vi "DblMonoPMDCurrentScanSM correction.vi"() -> ()   [LabVIEW 2009]
uses:
  <vilib>/DAQmx/create/channels.llb/DAQmx Create Channel (AI-Voltage-Basic).vi
  <vilib>/DAQmx/create/channels.llb/DAQmx Create Channel (AO-Voltage-Basic).vi
  <vilib>/DAQmx/write.llb/DAQmx Write (Analog DBL 1Chan 1Samp).vi
  <vilib>/DAQmx/read.llb/DAQmx Read (Analog 1D DBL 1Chan NSamp).vi
  <vilib>/DAQmx/configure/timing.llb/DAQmx Timing (Sample Clock).vi
  <vilib>/DAQmx/read.llb/DAQmx Read (Analog 1D DBL NChan 1Samp).vi
  <vilib>/DAQmx/write.llb/DAQmx Write (Analog 2D DBL NChan NSamp).vi
  <vilib>/Utility/file.llb/Write To Spreadsheet File (DBL).vi
  <vilib>/Analysis/NI_AALBase.lvlib
panel:
  in  "Volts/pixel":dbl
  out "Xin":dbl
  out "Yin":dbl
  in  "Correction":dbl[][](array[numeric])
  in  "Scan mirrors out":tag
  in  "Scan Mirrors in":tag
  in  "Voltage B":dbl min=-10.0 max=10.0 step=0.1 format="%0.2f"
  in  "Voltage A":dbl min=-10.0 max=10.0 step=0.1 format="%0.2f"
  in  "Output B":tag="Dev1/ao3"
  in  "Output A":tag="Dev1/ao2"
  in  "Input Channel":tag="Dev1/ai6"
  in  "Current":bool
  in  "Power":bool=TRUE
  out "ScanGraph":cluster{dbl[], dbl[]}(graph)
  in  "Sensitivity":dbl=1e-09 caption="(A/V)" format="%#_6p"
  out "Readout":dbl=-2.45576047e-07 format="%^#_9e"
  in  "Scan Save Path":path
  in  "On":bool=TRUE
  out "Waveform Chart":dbl(graph)=-2.45576047e-07
  in  "Save":bool=TRUE
  in  "Exit":bool
  in  "STOP":bool
  in  "Step Time (sec)":dbl=1.0 min=0.001 max=300.0 step=0.001 format="%.3f"
  in  "Step Size (nm)":dbl=1.0 min=0.1 max=100.0 step=0.1 format="%.1f"
  in  "End":dbl=800.0 min=0.0 max=2000.0 step=0.1 format="%.1f"
  in  "Start":dbl=400.0 min=0.0 max=2000.0 step=0.1 format="%.1f"
  in  "Scan":bool
  in  "Up":bool=TRUE caption="Down"
  in  "Increment (nm)":dbl=10.0 min=0.1 max=2000.0 step=0.1 format="%.1f"
  in  "PMD Settings":T1={"Beam Diameter (mm)"=4.0, "BWIn"=0, "Averaging Rate"=300, "Auto Range"=TRUE} {"Averaging Rate" min=33 max=5000 step=1; "BWIn" items=["HIGH", "LOW"]; "Beam Diameter (mm)" min=1.0 max=9.0 step=0.5}
  in  "Step":bool
  out "Busy":bool=TRUE
  in  "Send Command":bool
  in  "Command":u16(ring)=1 items=["nm", "goto", "nm/min", "VIS grating", "IR grating"]
  in  "Wavelength (nm)":dbl=500.0 min=0.0 max=2000.0 step=0.1 format="%.1f"
  in  "Scan Speed (nm/min)":dbl=100.0 min=1.0 max=500.0 step=0.1 format="%.1f"
  out "Done?":string="   ..."
  in  "Send Question":bool
  in  "Ask?":u16(ring) items=["?nm", "?nm/min", "?grating", "?turret", "?gratings"]
  in  "Zero?":bool
  out "PM Error log":string="-222,\"Data out of range\"\n-222,\"Data out of range\"\n-222,\"Data out of range\"\n-222,\"Data out of range\"\n-222,\"Data out of range\"\n-222,\"Data out of range\"\n-222,\"Data out of range\"\n-222,\"Data out of range\"\n-222,\"Data out of range\"\n-222,\"Data out of range\"\n-222,\"Data out of range\"\n-222,\"Data out of range\"\n-222,\"Data out of range\"\n-222,\"Data out of range\"\n-222,\"Data out of range\"\n-222,\"Data out of range\"\n-222,\"Data out of range\"\n-222,\"Data out of range\"\n-222,\"Data out of range\"\n-222,\"Data out of range\"\n-222,\"Data out of range\"\n-222,\"Data out of range\"\n-222,\"Data out of range\"\n-222,\"Data out of range\"\n-222,\"Data out of range\"\n-222,\"Data out of range\"\n-222,\"Data out of range\"\n-222,\"Data out of range\"\n-222,\"Data out of range\"\n-222,\"Data out of range\"\n-222,\"Data out of range\"\n-222,\"Data out of range\"\n-222,\"Data out of range\"\n-222,\"Data out of range\"\n-222,\"Data out of range\"\n-222,\"Data out of range\"\n-222,\"Data out of range\"\n-222,\"Data out of range\"\n-222,\"Data out of range\"\n-222,\"Data out of range\"\n-222,\"Data out of range\"\n-222,\"Data out of range\"\n-222,\"Data out of range\"\n-222,\"Data out of range\"\n-222,\"Data out of range\"\n-222,\"Data out of range\"\n-222,\"Data out of range\"\n-222,\"Data out of range\"\n-222,\"Data out of range\"\n-222,\"Data out of range\"\n-222,\"Data out of range\"\n-222,\"Data out of range\"\n-222,\"Data out of range\"\n-222,\"Data out of range\"\n-222,\"Data out of range\"\n-222,\"Data out of range\"\n-222,\"Data out of range\"\n-222,\"Data out of range\"\n-222,\"Data out of range\"\n-222,\"Data out of range\"\n-222,\"Data out of range\"\n-222,\"Data out of range\"\n-222,\"Data out of range\"\n-222,\"Data out of range\"\n-222,\"Data out of range\"\n-222,\"Data out of range\"\n-222,\"Data out of range\"\n-222,\"Data out of range\"\n-222,\"Data out of range\"\n-222,\"Data out of range\"\n-222,\"Data out of range\"\n-222,\"Data out of range\"\n-222,\"Data out of range\"\n-222,\"Data out of range\"\n-222,\"Data out of range\"\n-222,\"Data out of range\"\n-222,\"Data out of range\"\n-222,\"Data out of range\"\n-222,\"Data out of range\"\n-222,\"Data out of range\"\n-222,\"Data out of range\"\n-222,\"Data out of range\"\n-222,\"Data out of range\"\n-222,\"Data out of range\"\n-222,\"Data out of range\"\n-222,\"Data out of range\"\n-222,\"Data out of range\"\n-222,\"Data out of range\"\n-222,\"Data out of range\"\n-222,\"Data out of range\"\n-222,\"Data out of range\"\n-222,\"Data out of range\"\n-222,\"Data out of range\"\n-222,\"Data out of range\"\n-222,\"Data out of range\"\n-222,\"Data out of range\"\n-222,\"Data out of range\"\n-222,\"Data out of range\"\n-222,\"Data out of range\"\n-222,\"Data out of range\"\n-222,\"Data out of range\"\n-222,\"Data out of range\"\n-222,\"Data out of range\"\n-222,\"Data out of range\"\n-222,\"Data out of range\"\n-222,\"Data out of range\"\n-222,\"Data out of range\"\n-222,\"Data out of range\"\n-222,\"Data out of range\"\n-222,\"Data out of range\"\n-222,\"Data out of range\"\n-222,\"Data out of range\"\n-222,\"Data out of range\"\n-222,\"Data out of range\"\n-222,\"Data out of range\"\n-222,\"Data out of range\"\n-222,\"Data out of range\"\n-222,\"Data out of range\"\n-222,\"Data out of range\"\n-222,\"Data out of range\"\n-222,\"Data out of range\"\n-222,\"Data out of range\"\n-222,\"Data out of range\"\n-222,\"Data out of range\"\n-222,\"Data out of range\"\n-222,\"Data out of range\"\n-222,\"Data out of range\"\n-222,\"Data out of range\"\n-222,\"Data out of range\"\n-222,\"Data out of range\"\n-222,\"Data out of range\"\n-222,\"Data out of range\"\n-222,\"Data out of range\"\n-222,\"Data out of range\"\n-222,\"Data out of range\"\n-222,\"Data out of range\"\n-222,\"Data out of range\"\n-222,\"Data out of range\"\n-222,\"Data out of range\"\n-222,\"Data out of range\"\n-222,\"Data out of range\"\n-222,\"Data out of range\"\n-222,\"Data out of range\"\n-222,\"Data out of range\"\n-222,\"Data out of range\"\n-222,\"Data out of range\"\n-222,\"Data out of range\"\n-222,\"Data out of range\"\n-222,\"Data out of range\"\n-222,\"Data out of range\"\n-222,\"Data out of range\"\n-222,\"Data out of range\"\n-222,\"Data out of range\"\n-222,\"Data out of range\"\n-222,\"Data out of range\"\n-222,\"Data out of range\"\n-222,\"Data out of range\"\n-222,\"Data out of range\"\n-222,\"Data out of range\"\n-222,\"Data out of range\"\n-222,\"Data out of range\"\n-222,\"Data out of range\"\n-222,\"Data out of range\"\n-222,\"Data out of range\"\n-222,\"Data out of range\"\n-222,\"Data out of range\"\n-222,\"Data out of range\"\n-222,\"Data out of range\"\n-222,\"Data out of range\"\n-222,\"Data out of range\"\n-222,\"Data out of range\"\n-222,\"Data out of range\"\n-222,\"Data out of range\"\n-222,\"Data out of range\"\n-222,\"Data out of range\"\n-222,\"Data out of range\"\n-222,\"Data out of range\"\n-222,\"Data out of range\"\n-222,\"Data out of range\"\n-222,\"Data out of range\"\n-222,\"Data out of range\"\n-222,\"Data out of range\"\n-222,\"Data out of range\"\n-222,\"Data out of range\"\n-222,\"Data out of range\"\n-222,\"Data out of range\"\n-222,\"Data out of range\"\n-222,\"Data out of range\"\n-222,\"Data out of range\"\n-222,\"Data out of range\"\n-222,\"Data out of range\"\n-222,\"Data out of range\"\n-222,\"Data out of range\"\n-222,\"Data out of range\"\n-222,\"Data out of range\"\n-222,\"Data out of range\"\n-222,\"Data out of range\"\n-222,\"Data out of range\"\n-222,\"Data out of range\"\n-222,\"Data out of range\"\n-222,\"Data out of range\"\n-222,\"Data out of range\"\n-222,\"Data out of range\"\n-222,\"Data out of range\"\n-222,\"Data out of range\"\n-222,\"Data out of range\"\n-222,\"Data out of range\"\n-222,\"Data out of range\"\n-222,\"Data out of range\"\n-222,\"Data out of range\"\n-222,\"Data out of range\"\n-222,\"Data out of range\"\n-222,\"Data out of range\"\n-222,\"Data out of range\"\n-222,\"Data out of range\"\n-222,\"Data out of range\"\n-222,\"Data out of range\"\n-222,\"Data out of range\"\n-222,\"Data out of range\"\n-222,\"Data out of range\"\n-222,\"Data out of range\"\n-222,\"Data out of range\"\n-222,\"Data out of range\"\n-222,\"Data out of range\"\n-222,\"Data out of range\"\n-222,\"Data out of range\"\n-222,\"Data out of range\"\n-222,\"Data out of range\"\n-222,\"Data out of range\"\n-222,\"Data out of range\"\n-222,\"Data out of range\"\n-222,\"Data out of range\"\n-222,\"Data out of range\"\n-222,\"Data out of range\"\n-222,\"Data out of range\"\n-222,\"Data out of range\"\n-222,\"Data out of range\"\n-222,\"Data out of range\"\n-222,\"Data out of range\"\n-222,\"Data out of range\"\n-222,\"Data out of range\"\n-222,\"Data out of range\"\n-222,\"Data out of range\"\n-222,\"Data out of range\"\n-222,\"Data out of range\"\n-222,\"Data out of range\"\n-222,\"Data out of range\"\n-222,\"Data out of range\"\n-222,\"Data out of range\"\n-222,\"Data out of range\"\n-222,\"Data out of range\"\n-222,\"Data out of range\"\n-222,\"Data out of range\"\n-222,\"Data out of range\"\n-222,\"Data out of range\"\n-222,\"Data out of range\"\n-222,\"Data out of range\"\n-222,\"Data out of range\"\n-222,\"Data out of range\"\n-222,\"Data out of range\"\n-222,\"Data out of range\"\n-222,\"Data out of range\"\n-222,\"Data out of range\"\n-222,\"Data out of range\"\n-222,\"Data out of range\"\n-222,\"Data out of range\"\n-222,\"Data out of range\"\n-222,\"Data out of range\"\n-222,\"Data out of range\"\n-222,\"Data out of range\"\n-222,\"Data out of range\"\n-222,\"Data out of range\"\n-222,\"Data out of range\"\n-222,\"Data out of range\"\n-222,\"Data out of range\"\n-222,\"Data out of range\"\n-222,\"Data out of range\"\n-222,\"Data out of range\"\n-222,\"Data out of range\"\n-222,\"Data out of range\"\n-222,\"Data out of range\"\n-222,\"Data out of range\"\n-222,\"Data out of range\"\n-222,\"Data out of range\"\n-222,\"Data out of range\"\n-222,\"Data out of range\"\n-222,\"Data out of range\"\n-222,\"Data out of range\"\n-222,\"Data out of range\"\n-222,\"Data out of range\"\n-222,\"Data out of range\"\n-222,\"Data out of range\"\n-222,\"Data out of range\"\n-222,\"Data out of range\"\n-222,\"Data out of range\"\n-222,\"Data out of range\"\n-222,\"Data out of range\"\n-222,\"Data out of range\"\n-222,\"Data out of range\"\n-222,\"Data out of range\"\n-222,\"Data out of range\"\n-222,\"Data out of range\"\n-222,\"Data out of range\"\n-222,\"Data out of range\"\n-222,\"Data out of range\"\n-222,\"Data out of range\"\n-222,\"Data out of range\"\n-222,\"Data out of range\"\n-222,\"Data out of range\"\n-222,\"Data out of range\"\n-222,\"Data out of range\"\n-222,\"Data out of range\"\n-222,\"Data out of range\"\n-222,\"Data out of range\"\n-222,\"Data out of range\"\n-222,\"Data out of range\"\n-222,\"Data out of range\"\n-222,\"Data out of range\"\n-222,\"Data out of range\"\n-222,\"Data out of range\"\n-222,\"Data out of range\"\n-222,\"Data out of range\"\n-222,\"Data out of range\"\n-222,\"Data out of range\"\n-222,\"Data out of range\"\n-222,\"Data out of range\"\n-222,\"Data out of range\"\n-222,\"Data out of range\"\n-222,\"Data out of range\"\n-222,\"Data out of range\"\n-222,\"Data out of range\"\n-222,\"Data out of range\"\n-222,\"Data out of range\"\n-222,\"Data out of range\"\n-222,\"Data out of range\"\n-222,\"Data out of range\"\n-222,\"Data out of range\"\n-222,\"Data out of range\"\n-222,\"Data out of range\"\n-222,\"Data out of range\"\n-222,\"Data out of range\"\n-222,\"Data out of range\"\n-222,\"Data out of range\"\n-222,\"Data out of range\"\n-222,\"Data out of range\"\n-222,\"Data out of range\"\n-222,\"Data out of range\"\n-222,\"Data out of range\"\n-222,\"Data out of range\"\n-222,\"Data out of range\"\n-222,\"Data out of range\"\n-222,\"Data out of range\"\n-222,\"Data out of range\"\n-222,\"Data out of range\"\n-222,\"Data out of range\"\n-222,\"Data out of range\"\n-222,\"Data out of range\"\n-222,\"Data out of range\"\n-222,\"Data out of range\"\n-222,\"Data out of range\"\n-222,\"Data out of range\"\n-222,\"Data out of range\"\n-222,\"Data out of range\"\n-222,\"Data out of range\"\n-222,\"Data out of range\"\n-222,\"Data out of range\"\n-222,\"Data out of range\"\n-222,\"Data out of range\"\n-222,\"Data out of range\"\n-222,\"Data out of range\"\n-222,\"Data out of range\"\n-222,\"Data out of range\"\n-222,\"Data out of range\"\n-222,\"Data out of range\"\n-222,\"Data out of range\"\n-222,\"Data out of range\"\n-222,\"Data out of range\"\n-222,\"Data out of range\"\n-222,\"Data out of range\"\n-222,\"Data out of range\"\n-222,\"Data out of range\"\n-222,\"Data out of range\"\n-222,\"Data out of range\"\n-222,\"Data out of range\"\n-222,\"Data out of range\"\n-222,\"Data out of range\"\n-222,\"Data out of range\"\n-222,\"Data out of range\"\n-222,\"Data out of range\"\n-222,\"Data out of range\"\n-222,\"Data out of range\"\n-222,\"Data out of range\"\n-222,\"Data out of range\"\n-222,\"Data out of range\"\n-222,\"Data out of range\"\n-222,\"Data out of range\"\n-222,\"Data out of range\"\n-222,\"Data out of range\"\n-222,\"Data out of range\"\n-222,\"Data out of range\"\n-222,\"Data out of range\"\n-222,\"Data out of range\"\n-222,\"Data out of range\"\n-222,\"Data out of range\"\n-222,\"Data out of range\"\n-222,\"Data out of range\"\n-222,\"Data out of range\"\n-222,\"Data out of range\"\n-222,\"Data out of range\"\n-222,\"Data out of range\"\n-222,\"Data out of range\"\n-222,\"Data out of range\"\n-222,\"Data out of range\"\n-222,\"Data out of range\"\n-222,\"Data out of range\"\n-222,\"Data out of range\"\n-222,\"Data out of range\"\n-222,\"Data out of range\"\n-222,\"Data out of range\"\n-222,\"Data out of range\"\n-222,\"Data out of range\"\n-222,\"Data out of range\"\n-222,\"Data out of range\"\n-222,\"Data out of range\"\n-222,\"Data out of range\"\n-222,\"Data out of range\"\n-222,\"Data out of range\"\n-222,\"Data out of range\"\n-222,\"Data out of range\"\n-222,\"Data out of range\"\n-222,\"Data out of range\"\n-222,\"Data out of range\"\n-222,\"Data out of range\"\n-222,\"Data out of range\"\n-222,\"Data out of range\"\n-222,\"Data out of range\"\n-222,\"Data out of range\"\n-222,\"Data out of range\"\n-222,\"Data out of range\"\n-222,\"Data out of range\"\n-222,\"Data out of range\"\n-222,\"Data out of range\"\n-222,\"Data out of range\"\n-222,\"Data out of range\"\n-222,\"Data out of range\"\n-222,\"Data out of range\"\n-222,\"Data out of range\"\n-222,\"Data out of range\"\n-222,\"Data out of range\"\n-222,\"Data out of range\"\n-222,\"Data out of range\"\n-222,\"Data out of range\"\n-222,\"Data out of range\"\n-222,\"Data out of range\"\n-222,\"Data out of range\"\n-222,\"Data out of range\"\n-222,\"Data out of range\"\n-222,\"Data out of range\"\n-222,\"Data out of range\"\n-222,\"Data out of range\"\n-222,\"Data out of range\"\n-222,\"Data out of range\"\n-222,\"Data out of range\"\n-222,\"Data out of range\"\n-222,\"Data out of range\"\n-222,\"Data out of range\"\n-222,\"Data out of range\"\n-222,\"Data out of range\"\n-222,\"Data out of range\"\n-222,\"Data out of range\"\n-222,\"Data out of range\"\n-222,\"Data out of range\"\n-222,\"Data out of range\"\n-222,\"Data out of range\"\n-222,\"Data out of range\"\n-222,\"Data out of range\"\n-222,\"Data out of range\"\n-222,\"Data out of range\"\n-222,\"Data out of range\"\n-222,\"Data out of range\"\n-222,\"Data out of range\"\n-222,\"Data out of range\"\n-222,\"Data out of range\"\n-222,\"Data out of range\"\n-222,\"Data out of range\"\n-222,\"Data out of range\"\n-222,\"Data out of range\"\n-222,\"Data out of range\"\n-222,\"Data out of range\"\n-222,\"Data out of range\"\n-222,\"Data out of range\"\n-222,\"Data out of range\"\n-222,\"Data out of range\"\n-222,\"Data out of range\"\n-222,\"Data out of range\"\n-222,\"Data out of range\"\n-222,\"Data out of range\"\n-222,\"Data out of range\"\n-222,\"Data out of range\"\n-222,\"Data out of range\"\n-222,\"Data out of range\"\n-222,\"Data out of range\"\n-222,\"Data out of range\"\n-222,\"Data out of range\"\n-222,\"Data out of range\"\n-222,\"Data out of range\"\n-222,\"Data out of range\"\n-222,\"Data out of range\"\n-222,\"Data out of range\"\n-222,\"Data out of range\"\n-222,\"Data out of range\"\n-222,\"Data out of range\"\n-222,\"Data out of range\"\n-222,\"Data out of range\"\n-222,\"Data out of range\"\n-222,\"Data out of range\"\n-222,\"Data out of range\"\n-222,\"Data out of range\"\n-222,\"Data out of range\"\n-222,\"Data out of range\"\n-222,\"Data out of range\"\n-222,\"Data out of range\"\n-222,\"Data out of range\"\n-222,\"Data out of range\"\n-222,\"Data out of range\"\n-222,\"Data out of range\"\n-222,\"Data out of range\"\n-222,\"Data out of range\"\n-222,\"Data out of range\"\n-222,\"Data out of range\"\n-222,\"Data out of range\"\n-222,\"Data out of range\"\n-222,\"Data out of range\"\n-222,\"Data out of range\"\n-222,\"Data out of range\"\n-222,\"Data out of range\"\n-222,\"Data out of range\"\n-222,\"Data out of range\"\n-222,\"Data out of range\"\n-222,\"Data out of range\"\n-222,\"Data out of range\"\n-222,\"Data out of range\"\n-222,\"Data out of range\"\n-222,\"Data out of range\"\n-222,\"Data out of range\"\n-222,\"Data out of range\"\n-222,\"Data out of range\"\n-222,\"Data out of range\"\n-222,\"Data out of range\"\n-222,\"Data out of range\"\n-222,\"Data out of range\"\n-222,\"Data out of range\"\n-222,\"Data out of range\"\n-222,\"Data out of range\"\n-222,\"Data out of range\"\n-222,\"Data out of range\"\n-222,\"Data out of range\"\n-222,\"Data out of range\"\n-222,\"Data out of range\"\n-222,\"Data out of range\"\n-222,\"Data out of range\"\n-222,\"Data out of range\"\n-222,\"Data out of range\"\n-222,\"Data out of range\"\n-222,\"Data out of range\"\n-222,\"Data out of range\"\n-222,\"Data out of range\"\n-222,\"Data out of range\"\n-222,\"Data out of range\"\n-222,\"Data out of range\"\n-222,\"Data out of range\"\n-222,\"Data out of range\"\n-222,\"Data out of range\"\n-222,\"Data out of range\"\n-222,\"Data out of range\"\n-222,\"Data out of range\"\n-222,\"Data out of range\"\n-222,\"Data out of range\"\n-222,\"Data out of range\"\n-222,\"Data out of range\"\n-222,\"Data out of range\"\n-222,\"Data out of range\"\n-222,\"Data out of range\"\n-222,\"Data out of range\"\n-222,\"Data out of range\"\n-222,\"Data out of range\"\n-222,\"Data out of range\"\n-222,\"Data out of range\"\n-222,\"Data out of range\"\n-222,\"Data out of range\"\n-222,\"Data out of range\"\n-222,\"Data out of range\"\n-222,\"Data out of range\"\n-222,\"Data out of range\"\n-222,\"Data out of range\"\n-222,\"Data out of range\"\n-222,\"Data out of range\"\n-222,\"Data out of range\"\n-222,\"Data out of range\"\n-222,\"Data out of range\"\n-222,\"Data out of range\"\n-222,\"Data out of range\"\n-222,\"Data out of range\"\n-222,\"Data out of range\"\n-222,\"Data out of range\"\n-222,\"Data out of range\"\n-222,\"Data out of range\"\n-222,\"Data out of range\"\n-222,\"Data out of range\"\n-222,\"Data out of range\"\n-222,\"Data out of range\"\n-222,\"Data out of range\"\n-222,\"Data out of range\"\n-222,\"Data out of range\"\n-222,\"Data out of range\"\n-222,\"Data out of range\"\n-222,\"Data out of range\"\n-222,\"Data out of range\"\n-222,\"Data out of range\"\n-222,\"Data out of range\"\n-222,\"Data out of range\"\n-222,\"Data out of range\"\n-222,\"Data out of range\"\n-222,\"Data out of range\"\n-222,\"Data out of range\"\n-222,\"Data out of range\"\n-222,\"Data out of range\"\n-222,\"Data out of range\"\n-222,\"Data out of range\"\n-222,\"Data out of range\"\n-222,\"Data out of range\"\n-222,\"Data out of range\"\n-222,\"Data out of range\"\n-222,\"Data out of range\"\n-222,\"Data out of range\"\n-222,\"Data out of range\"\n-222,\"Data out of range\"\n-222,\"Data out of range\"\n-222,\"Data out of range\"\n-222,\"Data out of range\"\n-222,\"Data out of range\"\n-222,\"Data out of range\"\n-222,\"Data out of range\"\n-222,\"Data out of range\"\n-222,\"Data out of range\"\n-222,\"Data out of range\"\n-222,\"Data out of range\"\n-222,\"Data out of range\"\n-222,\"Data out of range\"\n-222,\"Data out of range\"\n-222,\"Data out of range\"\n-222,\"Data out of range\"\n-222,\"Data out of range\"\n-222,\"Data out of range\"\n-222,\"Data out of range\"\n-222,\"Data out of range\"\n-222,\"Data out of range\"\n-222,\"Data out of range\"\n-222,\"Data out of range\"\n-222,\"Data out of range\"\n-222,\"Data out of range\"\n-222,\"Data out of range\"\n-222,\"Data out of range\"\n-222,\"Data out of range\"\n-222,\"Data out of range\"\n-222,\"Data out of range\"\n-222,\"Data out of range\"\n-222,\"Data out of range\"\n-222,\"Data out of range\"\n-222,\"Data out of range\"\n-222,\"Data out of range\"\n-222,\"Data out of range\"\n-222,\"Data out of range\"\n-222,\"Data out of range\"\n-222,\"Data out of range\"\n-222,\"Data out of range\"\n-222,\"Data out of range\"\n-222,\"Data out of range\"\n-222,\"Data out of range\"\n-222,\"Data out of range\"\n-222,\"Data out of range\"\n-222,\"Data out of range\"\n-222,\"Data out of range\"\n-222,\"Data out of range\"\n-222,\"Data out of range\"\n-222,\"Data out of range\"\n-222,\"Data out of range\"\n-222,\"Data out of range\"\n-222,\"Data out of range\"\n-222,\"Data out of range\"\n-222,\"Data out of range\"\n-222,\"Data out of range\"\n-222,\"Data out of range\"\n-222,\"Data out of range\"\n-222,\"Data out of range\"\n-222,\"Data out of range\"\n-222,\"Data out of range\"\n-222,\"Data out of range\"\n-222,\"Data out of range\"\n-222,\"Data out of range\"\n-222,\"Data out of range\"\n-222,\"Data out of range\"\n-222,\"Data out of range\"\n-222,\"Data out of range\"\n-222,\"Data out of range\"\n-222,\"Data out of range\"\n-222,\"Data out of range\"\n-222,\"Data out of range\"\n-222,\"Data out of range\"\n-222,\"Data out of range\"\n-222,\"Data out of range\"\n-222,\"Data out of range\"\n-222,\"Data out of range\"\n-222,\"Data out of range\"\n-222,\"Data out of range\"\n-222,\"Data out of range\"\n-222,\"Data out of range\"\n-222,\"Data out of range\"\n-222,\"Data out of range\"\n-222,\"Data out of range\"\n-222,\"Data out of range\"\n-222,\"Data out of range\"\n-222,\"Data out of range\"\n-222,\"Data out of range\"\n-222,\"Data out of range\"\n-222,\"Data out of range\"\n-222,\"Data out of range\"\n-222,\"Data out of range\"\n-222,\"Data out of range\"\n-222,\"Data out of range\"\n-222,\"Data out of range\"\n-222,\"Data out of range\"\n-222,\"Data out of range\"\n-222,\"Data out of range\"\n-222,\"Data out of range\"\n-222,\"Data out of range\"\n-222,\"Data out of range\"\n-222,\"Data out of range\"\n-222,\"Data out of range\"\n-222,\"Data out of range\"\n-222,\"Data out of range\"\n-222,\"Data out of range\"\n-222,\"Data out of range\"\n-222,\"Data out of range\"\n-222,\"Data out of range\"\n-222,\"Data out of range\"\n-222,\"Data out of range\"\n-222,\"Data out of range\"\n-222,\"Data out of range\"\n-222,\"Data out of range\"\n-222,\"Data out of range\"\n-222,\"Data out of range\"\n-222,\"Data out of range\"\n-222,\"Data out of range\"\n-222,\"Data out of range\"\n-222,\"Data out of range\"\n-222,\"Data out of range\"\n-222,\"Data out of range\"\n-222,\"Data out of range\"\n-222,\"Data out of range\"\n-222,\"Data out of range\"\n-222,\"Data out of range\"\n-222,\"Data out of range\"\n-222,\"Data out of range\"\n-222,\"Data out of range\"\n-222,\"Data out of range\"\n-222,\"Data out of range\"\n-222,\"Data out of range\"\n-222,\"Data out of range\"\n-222,\"Data out of range\"\n-222,\"Data out of range\"\n-222,\"Data out of range\"\n-222,\"Data out of range\"\n-222,\"Data out of range\"\n-222,\"Data out of range\"\n-222,\"Data out of range\"\n-222,\"Data out of range\"\n-222,\"Data out of range\"\n-222,\"Data out of range\"\n-222,\"Data out of range\"\n-222,\"Data out of range\"\n-222,\"Data out of range\"\n-222,\"Data out of range\"\n-222,\"Data out of range\"\n-222,\"Data out of range\"\n-222,\"Data out of range\"\n-222,\"Data out of range\"\n-222,\"Data out of range\"\n-222,\"Data out of range\"\n-222,\"Data out of range\"\n-222,\"Data out of range\"\n-222,\"Data out of range\"\n-222,\"Data out of range\"\n-222,\"Data out of range\"\n-222,\"Data out of range\"\n-222,\"Data out of range\"\n-222,\"Data out of range\"\n-222,\"Data out of range\"\n-222,\"Data out of range\"\n-222,\"Data out of range\"\n-222,\"Data out of range\"\n-222,\"Data out of range\"\n-222,\"Data out of range\"\n-222,\"Data out of range\"\n-222,\"Data out of range\"\n-222,\"Data out of range\"\n-222,\"Data out of range\"\n-222,\"Data out of range\"\n-222,\"Data out of range\"\n-222,\"Data out of range\"\n-222,\"Data out of range\"\n-222,\"Data out of range\"\n-222,\"Data out of range\"\n-222,\"Data out of range\"\n-222,\"Data out of range\"\n-222,\"Data out of range\"\n-222,\"Data out of range\"\n-222,\"Data out of range\"\n-222,\"Data out of range\"\n-222,\"Data out of range\"\n-222,\"Data out of range\"\n-222,\"Data out of range\"\n-222,\"Data out of range\"\n-222,\"Data out of range\"\n-222,\"Data out of range\"\n-222,\"Data out of range\"\n-222,\"Data out of range\"\n-222,\"Data out of range\"\n-222,\"Data out of range\"\n-222,\"Data out of range\"\n-222,\"Data out of range\"\n-222,\"Data out of range\"\n-222,\"Data out of range\"\n-222,\"Data out of range\"\n-222,\"Data out of range\"\n-222,\"Data out of range\"\n-222,\"Data out of range\"\n-222,\"Data out of range\"\n-222,\"Data out of range\"\n-222,\"Data out of range\"\n-222,\"Data out of range\"\n-222,\"Data out of range\"\n-222,\"Data out of range\"\n-222,\"Data out of range\"\n-222,\"Data out of range\"\n-222,\"Data out of range\"\n-222,\"Data out of range\"\n-222,\"Data out of range\"\n-222,\"Data out of range\"\n-222,\"Data out of range\"\n-222,\"Data out of range\"\n-222,\"Data out of range\"\n-222,\"Data out of range\"\n-222,\"Data out of range\"\n-222,\"Data out of range\"\n-222,\"Data out of range\"\n-222,\"Data out of range\"\n-222,\"Data out of range\"\n-222,\"Data out of range\"\n-222,\"Data out of range\"\n-222,\"Data out of range\"\n-222,\"Data out of range\"\n-222,\"Data out of range\"\n-222,\"Data out of range\"\n-222,\"Data out of range\"\n-222,\"Data out of range\"\n-222,\"Data out of range\"\n-222,\"Data out of range\"\n-222,\"Data out of range\"\n-222,\"Data out of range\"\n-222,\"Data out of range\"\n-222,\"Data out of range\"\n-222,\"Data out of range\"\n-222,\"Data out of range\"\n-222,\"Data out of range\"\n-222,\"Data out of range\"\n-222,\"Data out of range\"\n-222,\"Data out of range\"\n-222,\"Data out of range\"\n-222,\"Data out of range\"\n-222,\"Data out of range\"\n-222,\"Data out of range\"\n-222,\"Data out of range\"\n-222,\"Data out of range\"\n-222,\"Data out of range\"\n-222,\"Data out of range\"\n-222,\"Data out of range\"\n-222,\"Data out of range\"\n-222,\"Data out of range\"\n-222,\"Data out of range\"\n-222,\"Data out of range\"\n-222,\"Data out of range\"\n-222,\"Data out of range\"\n-222,\"Data out of range\"\n-222,\"Data out of range\"\n-222,\"Data out of range\"\n-222,\"Data out of range\"\n-222,\"Data out of range\"\n-222,\"Data out of range\"\n-222,\"Data out of range\"\n-222,\"Data out of range\"\n-222,\"Data out of range\"\n-222,\"Data out of range\"\n-222,\"Data out of range\"\n-222,\"Data out of range\"\n-222,\"Data out of range\"\n-222,\"Data out of range\"\n-222,\"Data out of range\"\n-222,\"Data out of range\"\n-222,\"Data out of range\"\n-222,\"Data out of range\"\n-222,\"Data out of range\"\n-222,\"Data out of range\"\n-222,\"Data out of range\"\n-222,\"Data out of range\"\n-222,\"Data out of range\"\n-222,\"Data out of range\"\n-222,\"Data out of range\"\n-222,\"Data out of range\"\n-222,\"Data out of range\"\n-222,\"Data out of range\"\n-222,\"Data out of range\"\n-222,\"Data out of range\"\n-222,\"Data out of range\"\n-222,\"Data out of range\"\n-222,\"Data out of range\"\n-222,\"Data out of range\"\n-222,\"Data out of range\"\n-222,\"Data out of range\"\n-222,\"Data out of range\"\n-222,\"Data out of range\"\n-222,\"Data out of range\"\n-222,\"Data out of range\"\n-222,\"Data out of range\"\n-222,\"Data out of range\"\n-222,\"Data out of range\"\n-222,\"Data out of range\"\n-222,\"Data out of range\"\n-222,\"Data out of range\"\n-222,\"Data out of range\"\n-222,\"Data out of range\"\n-222,\"Data out of range\"\n-222,\"Data out of range\"\n-222,\"Data out of range\"\n-222,\"Data out of range\"\n-222,\"Data out of range\"\n-222,\"Data out of range\"\n-222,\"Data out of range\"\n-222,\"Data out of range\"\n-222,\"Data out of range\"\n-222,\"Data out of range\"\n-222,\"Data out of range\"\n-222,\"Data out of range\"\n-222,\"Data out of range\"\n-222,\"Data out of range\"\n-222,\"Data out of range\"\n-222,\"Data out of range\"\n-222,\"Data out of range\"\n-222,\"Data out of range\"\n-222,\"Data out of range\"\n-222,\"Data out of range\"\n-222,\"Data out of range\"\n-222,\"Data out of range\"\n-222,\"Data out of range\"\n-222,\"Data out of range\"\n-222,\"Data out of range\"\n-222,\"Data out of range\"\n-222,\"Data out of range\"\n-222,\"Data out of range\"\n-222,\"Data out of range\"\n-222,\"Data out of range\"\n-222,\"Data out of range\"\n-222,\"Data out of range\"\n-222,\"Data out of range\"\n-222,\"Data out of range\"\n-222,\"Data out of range\"\n-222,\"Data out of range\"\n-222,\"Data out of range\"\n-222,\"Data out of range\"\n-222,\"Data out of range\"\n-222,\"Data out of range\"\n-222,\"Data out of range\"\n-222,\"Data out of range\"\n-222,\"Data out of range\"\n-222,\"Data out of range\"\n-222,\"Data out of range\"\n-222,\"Data out of range\"\n-222,\"Data out of range\"\n-222,\"Data out of range\"\n-222,\"Data out of range\"\n-222,\"Data out of range\"\n-222,\"Data out of range\"\n-222,\"Data out of range\"\n-222,\"Data out of range\"\n-222,\"Data out of range\"\n-222,\"Data out of range\"\n-222,\"Data out of range\"\n-222,\"Data out of range\"\n-222,\"Data out of range\"\n-222,\"Data out of range\"\n-222,\"Data out of range\"\n-222,\"Data out of range\"\n-222,\"Data out of range\"\n-222,\"Data out of range\"\n-222,\"Data out of range\"\n-222,\"Data out of range\"\n-222,\"Data out of range\"\n-222,\"Data out of range\"\n-222,\"Data out of range\"\n-222,\"Data out of range\"\n-222,\"Data out of range\"\n-222,\"Data out of range\"\n-222,\"Data out of range\"\n-222,\"Data out of range\"\n-222,\"Data out of range\"\n-222,\"Data out of range\"\n-222,\"Data out of range\"\n-222,\"Data out of range\"\n-222,\"Data out of range\"\n-222,\"Data out of range\"\n-222,\"Data out of range\"\n-222,\"Data out of range\"\n-222,\"Data out of range\"\n-222,\"Data out of range\"\n-222,\"Data out of range\"\n-222,\"Data out of range\"\n-222,\"Data out of range\"\n-222,\"Data out of range\"\n-222,\"Data out of range\"\n-222,\"Data out of range\"\n-222,\"Data out of range\"\n-222,\"Data out of range\"\n-222,\"Data out of range\"\n-222,\"Data out of range\"\n-222,\"Data out of range\"\n-222,\"Data out of range\"\n-222,\"Data out of range\"\n-222,\"Data out of range\"\n-222,\"Data out of range\"\n-222,\"Data out of range\"\n-222,\"Data out of range\"\n-222,\"Data out of range\"\n-222,\"Data out of range\"\n-222,\"Data out of range\"\n-222,\"Data out of range\"\n-222,\"Data out of range\"\n-222,\"Data out of range\"\n-222,\"Data out of range\"\n-222,\"Data out of range\"\n-222,\"Data out of range\"\n-222,\"Data out of range\"\n-222,\"Data out of range\"\n-222,\"Data out of range\"\n-222,\"Data out of range\"\n-222,\"Data out of range\"\n-222,\"Data out of range\"\n-222,\"Data out of range\"\n-222,\"Data out of range\"\n-222,\"Data out of range\"\n-222,\"Data out of range\"\n-222,\"Data out of range\"\n-222,\"Data out of range\"\n-222,\"Data out of range\"\n-222,\"Data out of range\"\n-222,\"Data out of range\"\n-222,\"Data out of range\"\n-222,\"Data out of range\"\n-222,\"Data out of range\"\n-222,\"Data out of range\"\n-222,\"Data out of range\"\n-222,\"Data out of range\"\n-222,\"Data out of range\"\n-222,\"Data out of range\"\n-222,\"Data out of range\"\n-222,\"Data out of range\"\n-222,\"Data out of range\"\n-222,\"Data out of range\"\n-222,\"Data out of range\"\n-222,\"Data out of range\"\n-222,\"Data out of range\"\n-222,\"Data out of range\"\n-222,\"Data out of range\"\n-222,\"Data out of range\"\n-222,\"Data out of range\"\n-222,\"Data out of range\"\n-222,\"Data out of range\"\n-222,\"Data out of range\"\n-222,\"Data out of range\"\n-222,\"Data out of range\"\n-222,\"Data out of range\"\n-222,\"Data out of range\"\n-222,\"Data out of range\"\n-222,\"Data out of range\"\n-222,\"Data out of range\"\n-222,\"Data out of range\"\n-222,\"Data out of range\"\n-222,\"Data out of range\"\n-222,\"Data out of range\"\n-222,\"Data out of range\"\n-222,\"Data out of range\"\n-222,\"Data out of range\"\n-222,\"Data out of range\"\n-222,\"Data out of range\"\n-222,\"Data out of range\"\n-222,\"Data out of range\"\n-222,\"Data out of range\"\n-222,\"Data out of range\"\n-222,\"Data out of range\"\n-222,\"Data out of range\"\n-222,\"Data out of range\"\n-222,\"Data out of range\"\n-222,\"Data out of range\"\n-222,\"Data out of range\"\n-222,\"Data out of range\"\n-222,\"Data out of range\"\n-222,\"Data out of range\"\n-222,\"Data out of range\"\n-222,\"Data out of range\"\n-222,\"Data out of range\"\n-222,\"Data out of range\"\n-222,\"Data out of range\"\n-222,\"Data out of range\"\n-222,\"Data out of range\"\n-222,\"Data out of range\"\n-222,\"Data out of range\"\n-222,\"Data out of range\"\n-222,\"Data out of range\"\n-222,\"Data out of range\"\n-222,\"Data out of range\"\n-222,\"Data out of range\"\n-222,\"Data out of range\"\n-222,\"Data out of range\"\n-222,\"Data out of range\"\n-222,\"Data out of range\"\n-222,\"Data out of range\"\n-222,\"Data out of range\"\n-222,\"Data out of range\"\n-222,\"Data out of range\"\n-222,\"Data out of range\"\n-222,\"Data out of range\"\n-222,\"Data out of range\"\n-222,\"Data out of range\"\n-222,\"Data out of range\"\n-222,\"Data out of range\"\n-222,\"Data out of range\"\n-222,\"Data out of range\"\n-222,\"Data out of range\"\n-222,\"Data out of range\"\n-222,\"Data out of range\"\n-222,\"Data out of range\"\n-222,\"Data out of range\"\n-222,\"Data out of range\"\n-222,\"Data out of range\"\n-222,\"Data out of range\"\n-222,\"Data out of range\"\n-222,\"Data out of range\"\n-222,\"Data out of range\"\n-222,\"Data out of range\"\n-222,\"Data out of range\"\n-222,\"Data out of range\"\n-222,\"Data out of range\"\n-222,\"Data out of range\"\n-222,\"Data out of range\"\n-222,\"Data out of range\"\n-222,\"Data out of range\"\n-222,\"Data out of range\"\n-222,\"Data out of range\"\n-222,\"Data out of range\"\n-222,\"Data out of range\"\n-222,\"Data out of range\"\n-222,\"Data out of range\"\n-222,\"Data out of range\"\n-222,\"Data out of range\"\n-222,\"Data out of range\"\n-222,\"Data out of range\"\n-222,\"Data out of range\"\n-222,\"Data out of range\"\n-222,\"Data out of range\"\n-222,\"Data out of range\"\n-222,\"Data out of range\"\n-222,\"Data out of range\"\n-222,\"Data out of range\"\n-222,\"Data out of range\"\n-222,\"Data out of range\"\n-222,\"Data out of range\"\n-222,\"Data out of range\"\n-222,\"Data out of range\"\n-222,\"Data out of range\"\n-222,\"Data out of range\"\n-222,\"Data out of range\"\n-222,\"Data out of range\"\n-222,\"Data out of range\"\n-222,\"Data out of range\"\n-222,\"Data out of range\"\n-222,\"Data out of range\"\n-222,\"Data out of range\"\n-222,\"Data out of range\"\n-222,\"Data out of range\"\n-222,\"Data out of range\"\n-222,\"Data out of range\"\n-222,\"Data out of range\"\n-222,\"Data out of range\"\n-222,\"Data out of range\"\n-222,\"Data out of range\"\n-222,\"Data out of range\"\n-222,\"Data out of range\"\n-222,\"Data out of range\"\n-222,\"Data out of range\"\n-222,\"Data out of range\"\n-222,\"Data out of range\"\n-222,\"Data out of range\"\n-222,\"Data out of range\"\n-222,\"Data out of range\"\n-222,\"Data out of range\"\n-222,\"Data out of range\"\n-222,\"Data out of range\"\n-222,\"Data out of range\"\n-222,\"Data out of range\"\n-222,\"Data out of range\"\n-222,\"Data out of range\"\n-222,\"Data out of range\"\n-222,\"Data out of range\"\n-222,\"Data out of range\"\n-222,\"Data out of range\"\n-222,\"Data out of range\"\n-222,\"Data out of range\"\n-222,\"Data out of range\"\n-222,\"Data out of range\"\n-222,\"Data out of range\"\n-222,\"Data out of range\"\n-222,\"Data out of range\"\n-222,\"Data out of range\"\n-222,\"Data out of range\"\n-222,\"Data out of range\"\n-222,\"Data out of range\"\n-222,\"Data out of range\"\n-222,\"Data out of range\"\n-222,\"Data out of range\"\n-222,\"Data out of range\"\n-222,\"Data out of range\"\n-222,\"Data out of range\"\n-222,\"Data out of range\"\n-222,\"Data out of range\"\n-222,\"Data out of range\"\n-222,\"Data out of range\"\n-222,\"Data out of range\"\n-222,\"Data out of range\"\n-222,\"Data out of range\"\n-222,\"Data out of range\"\n-222,\"Data out of range\"\n-222,\"Data out of range\"\n-222,\"Data out of range\"\n-222,\"Data out of range\"\n-222,\"Data out of range\"\n-222,\"Data out of range\"\n-222,\"Data out of range\"\n-222,\"Data out of range\"\n-222,\"Data out of range\"\n-222,\"Data out of range\"\n-222,\"Data out of range\"\n-222,\"Data out of range\"\n-222,\"Data out of range\"\n-222,\"Data out of range\"\n-222,\"Data out of range\"\n-222,\"Data out of range\"\n-222,\"Data out of range\"\n-222,\"Data out of range\"\n-222,\"Data out of range\"\n-222,\"Data out of range\"\n-222,\"Data out of range\"\n-222,\"Data out of range\"\n-222,\"Data out of range\"\n-222,\"Data out of range\"\n-222,\"Data out of range\"\n-222,\"Data out of range\"\n-222,\"Data out of range\"\n-222,\"Data out of range\"\n-222,\"Data out of range\"\n-222,\"Data out of range\"\n-222,\"Data out of range\"\n-222,\"Data out of range\"\n-222,\"Data out of range\"\n-222,\"Data out of range\"\n-222,\"Data out of range\"\n-222,\"Data out of range\"\n-222,\"Data out of range\"\n-222,\"Data out of range\"\n-222,\"Data out of range\"\n-222,\"Data out of range\"\n-222,\"Data out of range\"\n-222,\"Data out of range\"\n-222,\"Data out of range\"\n-222,\"Data out of range\"\n-222,\"Data out of range\"\n-222,\"Data out of range\"\n-222,\"Data out of range\"\n-222,\"Data out of range\"\n-222,\"Data out of range\"\n-222,\"Data out of range\"\n-222,\"Data out of range\"\n-222,\"Data out of range\"\n-222,\"Data out of range\"\n-222,\"Data out of range\"\n-222,\"Data out of range\"\n-222,\"Data out of range\"\n-222,\"Data out of range\"\n-222,\"Data out of range\"\n-222,\"Data out of range\"\n-222,\"Data out of range\"\n-222,\"Data out of range\"\n-222,\"Data out of range\"\n-222,\"Data out of range\"\n-222,\"Data out of range\"\n-222,\"Data out of range\"\n-222,\"Data out of range\"\n-222,\"Data out of range\"\n-222,\"Data out of range\"\n-222,\"Data out of range\"\n-222,\"Data out of range\"\n-222,\"Data out of range\"\n-222,\"Data out of range\"\n-222,\"Data out of range\"\n-222,\"Data out of range\"\n-222,\"Data out of range\"\n-222,\"Data out of range\"\n-222,\"Data out of range\"\n-222,\"Data out of range\"\n-222,\"Data out of range\"\n-222,\"Data out of range\"\n-222,\"Data out of range\"\n-222,\"Data out of range\"\n-222,\"Data out of range\"\n-222,\"Data out of range\"\n-222,\"Data out of range\"\n-222,\"Data out of range\"\n-222,\"Data out of range\"\n-222,\"Data out of range\"\n-222,\"Data out of range\"\n-222,\"Data out of range\"\n-222,\"Data out of range\"\n-222,\"Data out of range\"\n-222,\"Data out of range\"\n-222,\"Data out of range\"\n-222,\"Data out of range\"\n-222,\"Data out of range\"\n-222,\"Data out of range\"\n-222,\"Data out of range\"\n-222,\"Data out of range\"\n-222,\"Data out of range\"\n-222,\"Data out of range\"\n-222,\"Data out of range\"\n-222,\"Data out of range\"\n-222,\"Data out of range\"\n-222,\"Data out of range\"\n-222,\"Data out of range\"\n-222,\"Data out of range\"\n-222,\"Data out of range\"\n-222,\"Data out of range\"\n-222,\"Data out of range\"\n-222,\"Data out of range\"\n-222,\"Data out of range\"\n-222,\"Data out of range\"\n-222,\"Data out of range\"\n-222,\"Data out of range\"\n-222,\"Data out of range\"\n-222,\"Data out of range\"\n-222,\"Data out of range\"\n-222,\"Data out of range\"\n-222,\"Data out of range\"\n-222,\"Data out of range\"\n-222,\"Data out of range\"\n-222,\"Data out of range\"\n-222,\"Data out of range\"\n-222,\"Data out of range\"\n-222,\"Data out of range\"\n-222,\"Data out of range\"\n-222,\"Data out of range\"\n-222,\"Data out of range\"\n-222,\"Data out of range\"\n-222,\"Data out of range\"\n-222,\"Data out of range\"\n-222,\"Data out of range\"\n-222,\"Data out of range\"\n-222,\"Data out of range\"\n-222,\"Data out of range\"\n-222,\"Data out of range\"\n-222,\"Data out of range\"\n-222,\"Data out of range\"\n-222,\"Data out of range\"\n-222,\"Data out of range\"\n-222,\"Data out of range\"\n-222,\"Data out of range\"\n-222,\"Data out of range\"\n-222,\"Data out of range\"\n-222,\"Data out of range\"\n-222,\"Data out of range\"\n-222,\"Data out of range\"\n-222,\"Data out of range\"\n-222,\"Data out of range\"\n-222,\"Data out of range\"\n-222,\"Data out of range\"\n-222,\"Data out of range\"\n-222,\"Data out of range\"\n-222,\"Data out of range\"\n-222,\"Data out of range\"\n-222,\"Data out of range\"\n-222,\"Data out of range\"\n-222,\"Data out of range\"\n-222,\"Data out of range\"\n-222,\"Data out of range\"\n-222,\"Data out of range\"\n-222,\"Data out of range\"\n-222,\"Data out of range\"\n-222,\"Data out of range\"\n-222,\"Data out of range\"\n-222,\"Data out of range\"\n-222,\"Data out of range\"\n-222,\"Data out of range\"\n-222,\"Data out of range\"\n-222,\"Data out of range\"\n-222,\"Data out of range\"\n-222,\"Data out of range\"\n-222,\"Data out of range\"\n-222,\"Data out of range\"\n-222,\"Data out of range\"\n-222,\"Data out of range\"\n-222,\"Data out of range\"\n-222,\"Data out of range\"\n-222,\"Data out of range\"\n-222,\"Data out of range\"\n-222,\"Data out of range\"\n-222,\"Data out of range\"\n-222,\"Data out of range\"\n-222,\"Data out of range\"\n-222,\"Data out of range\"\n-222,\"Data out of range\"\n-222,\"Data out of range\"\n-222,\"Data out of range\"\n-222,\"Data out of range\"\n-222,\"Data out of range\"\n-222,\"Data out of range\"\n-222,\"Data out of range\"\n-222,\"Data out of range\"\n-222,\"Data out of range\"\n-222,\"Data out of range\"\n-222,\"Data out of range\"\n-222,\"Data out of range\"\n-222,\"Data out of range\"\n-222,\"Data out of range\"\n-222,\"Data out of range\"\n-222,\"Data out of range\"\n-222,\"Data out of range\"\n-222,\"Data out of range\"\n-222,\"Data out of range\"\n-222,\"Data out of range\"\n-222,\"Data out of range\"\n-222,\"Data out of range\"\n-222,\"Data out of range\"\n-222,\"Data out of range\"\n-222,\"Data out of range\"\n-222,\"Data out of range\"\n-222,\"Data out of range\"\n-222,\"Data out of range\"\n-222,\"Data out of range\"\n-222,\"Data out of range\"\n-222,\"Data out of range\"\n-222,\"Data out of range\"\n-222,\"Data out of range\"\n-222,\"Data out of range\"\n-222,\"Data out of range\"\n-222,\"Data out of range\"\n-222,\"Data out of range\"\n-222,\"Data out of range\"\n-222,\"Data out of range\"\n-222,\"Data out of range\"\n-222,\"Data out of range\"\n-222,\"Data out of range\"\n-222,\"Data out of range\"\n-222,\"Data out of range\"\n-222,\"Data out of range\"\n-222,\"Data out of range\"\n-222,\"Data out of range\"\n-222,\"Data out of range\"\n-222,\"Data out of range\"\n-222,\"Data out of range\"\n-222,\"Data out of range\"\n-222,\"Data out of range\"\n-222,\"Data out of range\"\n-222,\"Data out of range\"\n-222,\"Data out of range\"\n-222,\"Data out of range\"\n-222,\"Data out of range\"\n-222,\"Data out of range\"\n-222,\"Data out of range\"\n-222,\"Data out of range\"\n-222,\"Data out of range\"\n-222,\"Data out of range\"\n-222,\"Data out of range\"\n-222,\"Data out of range\"\n-222,\"Data out of range\"\n-222,\"Data out of range\"\n-222,\"Data out of range\"\n-222,\"Data out of range\"\n-222,\"Data out of range\"\n-222,\"Data out of range\"\n-222,\"Data out of range\"\n-222,\"Data out of range\"\n-222,\"Data out of range\"\n-222,\"Data out of range\"\n-222,\"Data out of range\"\n-222,\"Data out of range\"\n-222,\"Data out of range\"\n-222,\"Data out of range\"\n-222,\"Data out of range\"\n-222,\"Data out of range\"\n-222,\"Data out of range\"\n-222,\"Data out of range\"\n-222,\"Data out of range\"\n-222,\"Data out of range\"\n-222,\"Data out of range\"\n-222,\"Data out of range\"\n-222,\"Data out of range\"\n-222,\"Data out of range\"\n-222,\"Data out of range\"\n-222,\"Data out of range\"\n-222,\"Data out of range\"\n-222,\"Data out of range\"\n-222,\"Data out of range\"\n-222,\"Data out of range\"\n-222,\"Data out of range\"\n-222,\"Data out of range\"\n-222,\"Data out of range\"\n-222,\"Data out of range\"\n-222,\"Data out of range\"\n-222,\"Data out of range\"\n-222,\"Data out of range\"\n-222,\"Data out of range\"\n-222,\"Data out of range\"\n-222,\"Data out of range\"\n-222,\"Data out of range\"\n-222,\"Data out of range\"\n-222,\"Data out of range\"\n-222,\"Data out of range\"\n-222,\"Data out of range\"\n-222,\"Data out of range\"\n-222,\"Data out of range\"\n-222,\"Data out of range\"\n-222,\"Data out of range\"\n-222,\"Data out of range\"\n-222,\"Data out of range\"\n-222,\"Data out of range\"\n-222,\"Data out of range\"\n-222,\"Data out of range\"\n-222,\"Data out of range\"\n-222,\"Data out of range\"\n-222,\"Data out of range\"\n-222,\"Data out of range\"\n-222,\"Data out of range\"\n-222,\"Data out of range\"\n-222,\"Data out of range\"\n-222,\"Data out of range\"\n-222,\"Data out of range\"\n-222,\"Data out of range\"\n-222,\"Data out of range\"\n-222,\"Data out of range\"\n-222,\"Data out of range\"\n-222,\"Data out of range\"\n-222,\"Data out of range\"\n-222,\"Data out of range\"\n-222,\"Data out of range\"\n-222,\"Data out of range\"\n-222,\"Data out of range\"\n-222,\"Data out of range\"\n-222,\"Data out of range\"\n-222,\"Data out of range\"\n-222,\"Data out of range\"\n-222,\"Data out of range\"\n-222,\"Data out of range\"\n-222,\"Data out of range\"\n-222,\"Data out of range\"\n-222,\"Data out of range\"\n-222,\"Data out of range\"\n-222,\"Data out of range\"\n-222,\"Data out of range\"\n-222,\"Data out of range\"\n-222,\"Data out of range\"\n-222,\"Data out of range\"\n-222,\"Data out of range\"\n-222,\"Data out of range\"\n-222,\"Data out of range\"\n-222,\"Data out of range\"\n-222,\"Data out of range\"\n-222,\"Data out of range\"\n-222,\"Data out of range\"\n-222,\"Data out of range\"\n-222,\"Data out of range\"\n-222,\"Data out of range\"\n-222,\"Data out of range\"\n-222,\"Data out of range\"\n-222,\"Data out of range\"\n-222,\"Data out of range\"\n-222,\"Data out of range\"\n-222,\"Data out of range\"\n-222,\"Data out of range\"\n-222,\"Data out of range\"\n-222,\"Data out of range\"\n-222,\"Data out of range\"\n-222,\"Data out of range\"\n-222,\"Data out of range\"\n-222,\"Data out of range\"\n-222,\"Data out of range\"\n-222,\"Data out of range\"\n-222,\"Data out of range\"\n-222,\"Data out of range\"\n-222,\"Data out of range\"\n-222,\"Data out of range\"\n-222,\"Data out of range\"\n-222,\"Data out of range\"\n-222,\"Data out of range\"\n-222,\"Data out of range\"\n-222,\"Data out of range\"\n-222,\"Data out of range\"\n-222,\"Data out of range\"\n-222,\"Data out of range\"\n-222,\"Data out of range\"\n-222,\"Data out of range\"\n-222,\"Data out of range\"\n-222,\"Data out of range\"\n-222,\"Data out of range\"\n-222,\"Data out of range\"\n-222,\"Data out of range\"\n-222,\"Data out of range\"\n-222,\"Data out of range\"\n-222,\"Data out of range\"\n-222,\"Data out of range\"\n-222,\"Data out of range\"\n-222,\"Data out of range\"\n-222,\"Data out of range\"\n-222,\"Data out of range\"\n-222,\"Data out of range\"\n-222,\"Data out of range\"\n-222,\"Data out of range\"\n-222,\"Data out of range\"\n-222,\"Data out of range\"\n-222,\"Data out of range\"\n-222,\"Data out of range\"\n-222,\"Data out of range\"\n-222,\"Data out of range\"\n-222,\"Data out of range\"\n-222,\"Data out of range\"\n-222,\"Data out of range\"\n-222,\"Data out of range\"\n-222,\"Data out of range\"\n-222,\"Data out of range\"\n-222,\"Data out of range\"\n-222,\"Data out of range\"\n-222,\"Data out of range\"\n-222,\"Data out of range\"\n-222,\"Data out of range\"\n-222,\"Data out of range\"\n-222,\"Data out of range\"\n-222,\"Data out of range\"\n-222,\"Data out of range\"\n-222,\"Data out of range\"\n-222,\"Data out of range\"\n-222,\"Data out of range\"\n-222,\"Data out of range\"\n-222,\"Data out of range\"\n-222,\"Data out of range\"\n-222,\"Data out of range\"\n-222,\"Data out of range\"\n-222,\"Data out of range\"\n-222,\"Data out of range\"\n-222,\"Data out of range\"\n-222,\"Data out of range\"\n-222,\"Data out of range\"\n-222,\"Data out of range\"\n-222,\"Data out of range\"\n-222,\"Data out of range\"\n-222,\"Data out of range\"\n-222,\"Data out of range\"\n-222,\"Data out of range\"\n-222,\"Data out of range\"\n-222,\"Data out of range\"\n-222,\"Data out of range\"\n-222,\"Data out of range\"\n-222,\"Data out of range\"\n-222,\"Data out of range\"\n-222,\"Data out of range\"\n-222,\"Data out of range\"\n-222,\"Data out of range\"\n-222,\"Data out of range\"\n-222,\"Data out of range\"\n-222,\"Data out of range\"\n-222,\"Data out of range\"\n-222,\"Data out of range\"\n-222,\"Data out of range\"\n-222,\"Data out of range\"\n-222,\"Data out of range\"\n-222,\"Data out of range\"\n-222,\"Data out of range\"\n-222,\"Data out of range\"\n-222,\"Data out of range\"\n-222,\"Data out of range\"\n-222,\"Data out of range\"\n-222,\"Data out of range\"\n-222,\"Data out of range\"\n-222,\"Data out of range\"\n-222,\"Data out of range\"\n-222,\"Data out of range\"\n-222,\"Data out of range\"\n-222,\"Data out of range\"\n-222,\"Data out of range\"\n-222,\"Data out of range\"\n-222,\"Data out of range\"\n-222,\"Data out of range\"\n-222,\"Data out of range\"\n-222,\"Data out of range\"\n-222,\"Data out of range\"\n-222,\"Data out of range\"\n-222,\"Data out of range\"\n-222,\"Data out of range\"\n-222,\"Data out of range\"\n-222,\"Data out of range\"\n-222,\"Data out of range\"\n-222,\"Data out of range\"\n-222,\"Data out of range\"\n-222,\"Data out of range\"\n-222,\"Data out of range\"\n-222,\"Data out of range\"\n-222,\"Data out of range\"\n-222,\"Data out of range\"\n-222,\"Data out of range\"\n-222,\"Data out of range\"\n-222,\"Data out of range\"\n-222,\"Data out of range\"\n-222,\"Data out of range\"\n-222,\"Data out of range\"\n-222,\"Data out of range\"\n-222,\"Data out of range\"\n-222,\"Data out of range\"\n-222,\"Data out of range\"\n-222,\"Data out of range\"\n-222,\"Data out of range\"\n-222,\"Data out of range\"\n-222,\"Data out of range\"\n-222,\"Data out of range\"\n-222,\"Data out of range\"\n-222,\"Data out of range\"\n-222,\"Data out of range\"\n-222,\"Data out of range\"\n-222,\"Data out of range\"\n-222,\"Data out of range\"\n-222,\"Data out of range\"\n-222,\"Data out of range\"\n-222,\"Data out of range\"\n-222,\"Data out of range\"\n-222,\"Data out of range\"\n-222,\"Data out of range\"\n-222,\"Data out of range\"\n-222,\"Data out of range\"\n-222,\"Data out of range\"\n-222,\"Data out of range\"\n-222,\"Data out of range\"\n-222,\"Data out of range\"\n-222,\"Data out of range\"\n-222,\"Data out of range\"\n-222,\"Data out of range\"\n-222,\"Data out of range\"\n-222,\"Data out of range\"\n-222,\"Data out of range\"\n-222,\"Data out of range\"\n-222,\"Data out of range\"\n-222,\"Data out of range\"\n-222,\"Data out of range\"\n-222,\"Data out of range\"\n-222,\"Data out of range\"\n-222,\"Data out of range\"\n-222,\"Data out of range\"\n-222,\"Data out of range\"\n-222,\"Data out of range\"\n-222,\"Data out of range\"\n-222,\"Data out of range\"\n-222,\"Data out of range\"\n-222,\"Data out of range\"\n-222,\"Data out of range\"\n-222,\"Data out of range\"\n-222,\"Data out of range\"\n-222,\"Data out of range\"\n-222,\"Data out of range\"\n-222,\"Data out of range\"\n-222,\"Data out of range\"\n-222,\"Data out of range\"\n-222,\"Data out of range\"\n-222,\"Data out of range\"\n-222,\"Data out of range\"\n-222,\"Data out of range\"\n-222,\"Data out of range\"\n-222,\"Data out of range\"\n-222,\"Data out of range\"\n-222,\"Data out of range\"\n-222,\"Data out of range\"\n-222,\"Data out of range\"\n-222,\"Data out of range\"\n-222,\"Data out of range\"\n-222,\"Data out of range\"\n-222,\"Data out of range\"\n-222,\"Data out of range\"\n-222,\"Data out of range\"\n-222,\"Data out of range\"\n-222,\"Data out of range\"\n-222,\"Data out of range\"\n-222,\"Data out of range\"\n-222,\"Data out of range\"\n-222,\"Data out of range\"\n-222,\"Data out of range\"\n-222,\"Data out of range\"\n-222,\"Data out of range\"\n-222,\"Data out of range\"\n-222,\"Data out of range\"\n-222,\"Data out of range\"\n-222,\"Data out of range\"\n-222,\"Data out of range\"\n-222,\"Data out of range\"\n-222,\"Data out of range\"\n-222,\"Data out of range\"\n-222,\"Data out of range\"\n-222,\"Data out of range\"\n-222,\"Data out of range\"\n-222,\"Data out of range\"\n-222,\"Data out of range\"\n-222,\"Data out of range\"\n-222,\"Data out of range\"\n-222,\"Data out of range\"\n-222,\"Data out of range\"\n-222,\"Data out of range\"\n-222,\"Data out of range\"\n-222,\"Data out of range\"\n-222,\"Data out of range\"\n-222,\"Data out of range\"\n-222,\"Data out of range\"\n-222,\"Data out of range\"\n-222,\"Data out of range\"\n-222,\"Data out of range\"\n-222,\"Data out of range\"\n-222,\"Data out of range\"\n-222,\"Data out of range\"\n-222,\"Data out of range\"\n-222,\"Data out of range\"\n-222,\"Data out of range\"\n-222,\"Data out of range\"\n-222,\"Data out of range\"\n-222,\"Data out of range\"\n-222,\"Data out of range\"\n-222,\"Data out of range\"\n-222,\"Data out of range\"\n-222,\"Data out of range\"\n-222,\"Data out of range\"\n-222,\"Data out of range\"\n-222,\"Data out of range\"\n-222,\"Data out of range\"\n-222,\"Data out of range\"\n-222,\"Data out of range\"\n-222,\"Data out of range\"\n-222,\"Data out of range\"\n-222,\"Data out of range\"\n-222,\"Data out of range\"\n-222,\"Data out of range\"\n-222,\"Data out of range\"\n-222,\"Data out of range\"\n-222,\"Data out of range\"\n-222,\"Data out of range\"\n-222,\"Data out of range\"\n-222,\"Data out of range\"\n-222,\"Data out of range\"\n-222,\"Data out of range\"\n-222,\"Data out of range\"\n-222,\"Data out of range\"\n-222,\"Data out of range\"\n-222,\"Data out of range\"\n-222,\"Data out of range\"\n-222,\"Data out of range\"\n-222,\"Data out of range\"\n-222,\"Data out of range\"\n-222,\"Data out of range\"\n-222,\"Data out of range\"\n-222,\"Data out of range\"\n-222,\"Data out of range\"\n-222,\"Data out of range\"\n-222,\"Data out of range\"\n-222,\"Data out of range\"\n-222,\"Data out of range\"\n-222,\"Data out of range\"\n-222,\"Data out of range\"\n-222,\"Data out of range\"\n-222,\"Data out of range\"\n-222,\"Data out of range\"\n-222,\"Data out of range\"\n-222,\"Data out of range\"\n-222,\"Data out of range\"\n-222,\"Data out of range\"\n-222,\"Data out of range\"\n-222,\"Data out of range\"\n-222,\"Data out of range\"\n-222,\"Data out of range\"\n-222,\"Data out of range\"\n-222,\"Data out of range\"\n-222,\"Data out of range\"\n-222,\"Data out of range\"\n-222,\"Data out of range\"\n-222,\"Data out of range\"\n-222,\"Data out of range\"\n-222,\"Data out of range\"\n-222,\"Data out of range\"\n-222,\"Data out of range\"\n-222,\"Data out of range\"\n-222,\"Data out of range\"\n-222,\"Data out of range\"\n-222,\"Data out of range\"\n-222,\"Data out of range\"\n-222,\"Data out of range\"\n-222,\"Data out of range\"\n-222,\"Data out of range\"\n-222,\"Data out of range\"\n-222,\"Data out of range\"\n-222,\"Data out of range\"\n-222,\"Data out of range\"\n-222,\"Data out of range\"\n-222,\"Data out of range\"\n-222,\"Data out of range\"\n-222,\"Data out of range\"\n-222,\"Data out of range\"\n-222,\"Data out of range\"\n-222,\"Data out of range\"\n-222,\"Data out of range\"\n-222,\"Data out of range\"\n-222,\"Data out of range\"\n-222,\"Data out of range\"\n-222,\"Data out of range\"\n-222,\"Data out of range\"\n-222,\"Data out of range\"\n-222,\"Data out of range\"\n-222,\"Data out of range\"\n-222,\"Data out of range\"\n-222,\"Data out of range\"\n-222,\"Data out of range\"\n-222,\"Data out of range\"\n-222,\"Data out of range\"\n-222,\"Data out of range\"\n-222,\"Data out of range\"\n-222,\"Data out of range\"\n-222,\"Data out of range\"\n-222,\"Data out of range\"\n-222,\"Data out of range\"\n-222,\"Data out of range\"\n-222,\"Data out of range\"\n-222,\"Data out of range\"\n-222,\"Data out of range\"\n-222,\"Data out of range\"\n-222,\"Data out of range\"\n-222,\"Data out of range\"\n-222,\"Data out of range\"\n-222,\"Data out of range\"\n-222,\"Data out of range\"\n-222,\"Data out of range\"\n-222,\"Data out of range\"\n-222,\"Data out of range\"\n-222,\"Data out of range\"\n-222,\"Data out of range\"\n-222,\"Data out of range\"\n-222,\"Data out of range\"\n-222,\"Data out of range\"\n-222,\"Data out of range\"\n-222,\"Data out of range\"\n-222,\"Data out of range\"\n-222,\"Data out of range\"\n-222,\"Data out of range\"\n-222,\"Data out of range\"\n-222,\"Data out of range\"\n-222,\"Data out of range\"\n-222,\"Data out of range\"\n-222,\"Data out of range\"\n-222,\"Data out of range\"\n-222,\"Data out of range\"\n-222,\"Data out of range\"\n-222,\"Data out of range\"\n-222,\"Data out of range\"\n-222,\"Data out of range\"\n-222,\"Data out of range\"\n-222,\"Data out of range\"\n-222,\"Data out of range\"\n-222,\"Data out of range\"\n-222,\"Data out of range\"\n-222,\"Data out of range\"\n-222,\"Data out of range\"\n-222,\"Data out of range\"\n-222,\"Data out of range\"\n-222,\"Data out of range\"\n-222,\"Data out of range\"\n-222,\"Data out of range\"\n-222,\"Data out of range\"\n-222,\"Data out of range\"\n-222,\"Data out of range\"\n-222,\"Data out of range\"\n-222,\"Data out of range\"\n-222,\"Data out of range\"\n-222,\"Data out of range\"\n-222,\"Data out of range\"\n-222,\"Data out of range\"\n-222,\"Data out of range\"\n-222,\"Data out of range\"\n-222,\"Data out of range\"\n-222,\"Data out of range\"\n-222,\"Data out of range\"\n-222,\"Data out of range\"\n-222,\"Data out of range\"\n-222,\"Data out of range\"\n-222,\"Data out of range\"\n-222,\"Data out of range\"\n-222,\"Data out of range\"\n-222,\"Data out of range\"\n-222,\"Data out of range\"\n-222,\"Data out of range\"\n-222,\"Data out of range\"\n-222,\"Data out of range\"\n-222,\"Data out of range\"\n-222,\"Data out of range\"\n-222,\"Data out of range\"\n-222,\"Data out of range\"\n-222,\"Data out of range\"\n-222,\"Data out of range\"\n-222,\"Data out of range\"\n-222,\"Data out of range\"\n-222,\"Data out of range\"\n-222,\"Data out of range\"\n-222,\"Data out of range\"\n-222,\"Data out of range\"\n-222,\"Data out of range\"\n-222,\"Data out of range\"\n-222,\"Data out of range\"\n-222,\"Data out of range\"\n-222,\"Data out of range\"\n-222,\"Data out of range\"\n-222,\"Data out of range\"\n-222,\"Data out of range\"\n-222,\"Data out of range\"\n-222,\"Data out of range\"\n-222,\"Data out of range\"\n-222,\"Data out of range\"\n-222,\"Data out of range\"\n-222,\"Data out of range\"\n-222,\"Data out of range\"\n-222,\"Data out of range\"\n-222,\"Data out of range\"\n-222,\"Data out of range\"\n-222,\"Data out of range\"\n-222,\"Data out of range\"\n-222,\"Data out of range\"\n-222,\"Data out of range\"\n-222,\"Data out of range\"\n-222,\"Data out of range\"\n-222,\"Data out of range\"\n-222,\"Data out of range\"\n-222,\"Data out of range\"\n-222,\"Data out of range\"\n-222,\"Data out of range\"\n-222,\"Data out of range\"\n-222,\"Data out of range\"\n-222,\"Data out of range\"\n-222,\"Data out of range\"\n-222,\"Data out of range\"\n-222,\"Data out of range\"\n-222,\"Data out of range\"\n-222,\"Data out of range\"\n-222,\"Data out of range\"\n-222,\"Data out of range\"\n-222,\"Data out of range\"\n-222,\"Data out of range\"\n-222,\"Data out of range\"\n-222,\"Data out of range\"\n-222,\"Data out of range\"\n-222,\"Data out of range\"\n-222,\"Data out of range\"\n-222,\"Data out of range\"\n-222,\"Data out of range\"\n-222,\"Data out of range\"\n-222,\"Data out of range\"\n-222,\"Data out of range\"\n-222,\"Data out of range\"\n-222,\"Data out of range\"\n-222,\"Data out of range\"\n-222,\"Data out of range\"\n-222,\"Data out of range\"\n-222,\"Data out of range\"\n-222,\"Data out of range\"\n-222,\"Data out of range\"\n-222,\"Data out of range\"\n-222,\"Data out of range\"\n-222,\"Data out of range\"\n-222,\"Data out of range\"\n-222,\"Data out of range\"\n-222,\"Data out of range\"\n-222,\"Data out of range\"\n-222,\"Data out of range\"\n-222,\"Data out of range\"\n-222,\"Data out of range\"\n-222,\"Data out of range\"\n-222,\"Data out of range\"\n-222,\"Data out of range\"\n-222,\"Data out of range\"\n-222,\"Data out of range\"\n-222,\"Data out of range\"\n-222,\"Data out of range\"\n-222,\"Data out of range\"\n-222,\"Data out of range\"\n-222,\"Data out of range\"\n-222,\"Data out of range\"\n-222,\"Data out of range\"\n-222,\"Data out of range\"\n-222,\"Data out of range\"\n-222,\"Data out of range\"\n-222,\"Data out of range\"\n-222,\"Data out of range\"\n-222,\"Data out of range\"\n-222,\"Data out of range\"\n-222,\"Data out of range\"\n-222,\"Data out of range\"\n-222,\"Data out of range\"\n-222,\"Data out of range\"\n-222,\"Data out of range\"\n-222,\"Data out of range\"\n-222,\"Data out of range\"\n-222,\"Data out of range\"\n-222,\"Data out of range\"\n-222,\"Data out of range\"\n-222,\"Data out of range\"\n-222,\"Data out of range\"\n-222,\"Data out of range\"\n-222,\"Data out of range\"\n-222,\"Data out of range\"\n-222,\"Data out of range\"\n-222,\"Data out of range\"\n-222,\"Data out of range\"\n-222,\"Data out of range\"\n-222,\"Data out of range\"\n-222,\"Data out of range\"\n-222,\"Data out of range\"\n-222,\"Data out of range\"\n-222,\"Data out of range\"\n-222,\"Data out of range\"\n-222,\"Data out of range\"\n-222,\"Data out of range\"\n-222,\"Data out of range\"\n-222,\"Data out of range\"\n-222,\"Data out of range\"\n-222,\"Data out of range\"\n-222,\"Data out of range\"\n-222,\"Data out of range\"\n-222,\"Data out of range\"\n-222,\"Data out of range\"\n-222,\"Data out of range\"\n-222,\"Data out of range\"\n-222,\"Data out of range\"\n-222,\"Data out of range\"\n-222,\"Data out of range\"\n-222,\"Data out of range\"\n-222,\"Data out of range\"\n-222,\"Data out of range\"\n-222,\"Data out of range\"\n-222,\"Data out of range\"\n-222,\"Data out of range\"\n-222,\"Data out of range\"\n-222,\"Data out of range\"\n-222,\"Data out of range\"\n-222,\"Data out of range\"\n-222,\"Data out of range\"\n-222,\"Data out of range\"\n-222,\"Data out of range\"\n-222,\"Data out of range\"\n-222,\"Data out of range\"\n-222,\"Data out of range\"\n-222,\"Data out of range\"\n-222,\"Data out of range\"\n-222,\"Data out of range\"\n-222,\"Data out of range\"\n-222,\"Data out of range\"\n-222,\"Data out of range\"\n-222,\"Data out of range\"\n-222,\"Data out of range\"\n-222,\"Data out of range\"\n-222,\"Data out of range\"\n-222,\"Data out of range\"\n-222,\"Data out of range\"\n-222,\"Data out of range\"\n-222,\"Data out of range\"\n-222,\"Data out of range\"\n-222,\"Data out of range\"\n-222,\"Data out of range\"\n-222,\"Data out of range\"\n-222,\"Data out of range\"\n-222,\"Data out of range\"\n-222,\"Data out of range\"\n-222,\"Data out of range\"\n-222,\"Data out of range\"\n-222,\"Data out of range\"\n-222,\"Data out of range\"\n-222,\"Data out of range\"\n-222,\"Data out of range\"\n-222,\"Data out of range\"\n-222,\"Data out of range\"\n-222,\"Data out of range\"\n-222,\"Data out of range\"\n-222,\"Data out of range\"\n-222,\"Data out of range\"\n-222,\"Data out of range\"\n-222,\"Data out of range\"\n-222,\"Data out of range\"\n-222,\"Data out of range\"\n-222,\"Data out of range\"\n-222,\"Data out of range\"\n-222,\"Data out of range\"\n-222,\"Data out of range\"\n-222,\"Data out of range\"\n-222,\"Data out of range\"\n-222,\"Data out of range\"\n-222,\"Data out of range\"\n-222,\"Data out of range\"\n-222,\"Data out of range\"\n-222,\"Data out of range\"\n-222,\"Data out of range\"\n-222,\"Data out of range\"\n-222,\"Data out of range\"\n-222,\"Data out of range\"\n-222,\"Data out of range\"\n-222,\"Data out of range\"\n-222,\"Data out of range\"\n-222,\"Data out of range\"\n-222,\"Data out of range\"\n-222,\"Data out of range\"\n-222,\"Data out of range\"\n-222,\"Data out of range\"\n-222,\"Data out of range\"\n-222,\"Data out of range\"\n-222,\"Data out of range\"\n-222,\"Data out of range\"\n-222,\"Data out of range\"\n-222,\"Data out of range\"\n-222,\"Data out of range\"\n-222,\"Data out of range\"\n-222,\"Data out of range\"\n-222,\"Data out of range\"\n-222,\"Data out of range\"\n-222,\"Data out of range\"\n-222,\"Data out of range\"\n-222,\"Data out of range\"\n-222,\"Data out of range\"\n-222,\"Data out of range\"\n-222,\"Data out of range\"\n-222,\"Data out of range\"\n-222,\"Data out of range\"\n-222,\"Data out of range\"\n-222,\"Data out of range\"\n-222,\"Data out of range\"\n-222,\"Data out of range\"\n-222,\"Data out of range\"\n-222,\"Data out of range\"\n-222,\"Data out of range\"\n-222,\"Data out of range\"\n-222,\"Data out of range\"\n-222,\"Data out of range\"\n-222,\"Data out of range\"\n-222,\"Data out of range\"\n-222,\"Data out of range\"\n-222,\"Data out of range\"\n-222,\"Data out of range\"\n-222,\"Data out of range\"\n-222,\"Data out of range\"\n-222,\"Data out of range\"\n-222,\"Data out of range\"\n-222,\"Data out of range\"\n-222,\"Data out of range\"\n-222,\"Data out of range\"\n-222,\"Data out of range\"\n-222,\"Data out of range\"\n-222,\"Data out of range\"\n-222,\"Data out of range\"\n-222,\"Data out of range\"\n-222,\"Data out of range\"\n-222,\"Data out of range\"\n-222,\"Data out of range\"\n-222,\"Data out of range\"\n-222,\"Data out of range\"\n-222,\"Data out of range\"\n-222,\"Data out of range\"\n-222,\"Data out of range\"\n-222,\"Data out of range\"\n-222,\"Data out of range\"\n-222,\"Data out of range\"\n-222,\"Data out of range\"\n-222,\"Data out of range\"\n-222,\"Data out of range\"\n-222,\"Data out of range\"\n-222,\"Data out of range\"\n-222,\"Data out of range\"\n-222,\"Data out of range\"\n-222,\"Data out of range\"\n-222,\"Data out of range\"\n-222,\"Data out of range\"\n-222,\"Data out of range\"\n-222,\"Data out of range\"\n-222,\"Data out of range\"\n-222,\"Data out of range\"\n-222,\"Data out of range\"\n-222,\"Data out of range\"\n-222,\"Data out of range\"\n-222,\"Data out of range\"\n-222,\"Data out of range\"\n-222,\"Data out of range\"\n-222,\"Data out of range\"\n-222,\"Data out of range\"\n-222,\"Data out of range\"\n-222,\"Data out of range\"\n-222,\"Data out of range\"\n-222,\"Data out of range\"\n-222,\"Data out of range\"\n-222,\"Data out of range\"\n-222,\"Data out of range\"\n-222,\"Data out of range\"\n-222,\"Data out of range\"\n-222,\"Data out of range\"\n-222,\"Data out of range\"\n-222,\"Data out of range\"\n-222,\"Data out of range\"\n-222,\"Data out of range\"\n-222,\"Data out of range\"\n-222,\"Data out of range\"\n-222,\"Data out of range\"\n-222,\"Data out of range\"\n-222,\"Data out of range\"\n-222,\"Data out of range\"\n-222,\"Data out of range\"\n-222,\"Data out of range\"\n-222,\"Data out of range\"\n-222,\"Data out of range\"\n-222,\"Data out of range\"\n-222,\"Data out of range\"\n-222,\"Data out of range\"\n-222,\"Data out of range\"\n-222,\"Data out of range\"\n-222,\"Data out of range\"\n-222,\"Data out of range\"\n-222,\"Data out of range\"\n-222,\"Data out of range\"\n-222,\"Data out of range\"\n-222,\"Data out of range\"\n-222,\"Data out of range\"\n-222,\"Data out of range\"\n-222,\"Data out of range\"\n-222,\"Data out of range\"\n-222,\"Data out of range\"\n-222,\"Data out of range\"\n-222,\"Data out of range\"\n-222,\"Data out of range\"\n-222,\"Data out of range\"\n-222,\"Data out of range\"\n-222,\"Data out of range\"\n-222,\"Data out of range\"\n-222,\"Data out of range\"\n-222,\"Data out of range\"\n-222,\"Data out of range\"\n-222,\"Data out of range\"\n-222,\"Data out of range\"\n-222,\"Data out of range\"\n-222,\"Data out of range\"\n-222,\"Data out of range\"\n-222,\"Data out of range\"\n-222,\"Data out of range\"\n-222,\"Data out of range\"\n-222,\"Data out of range\"\n-222,\"Data out of range\"\n-222,\"Data out of range\"\n-222,\"Data out of range\"\n-222,\"Data out of range\"\n-222,\"Data out of range\"\n-222,\"Data out of range\"\n-222,\"Data out of range\"\n-222,\"Data out of range\"\n-222,\"Data out of range\"\n-222,\"Data out of range\"\n-222,\"Data out of range\"\n-222,\"Data out of range\"\n-222,\"Data out of range\"\n-222,\"Data out of range\"\n-222,\"Data out of range\"\n-222,\"Data out of range\"\n-222,\"Data out of range\"\n-222,\"Data out of range\"\n-222,\"Data out of range\"\n-222,\"Data out of range\"\n-222,\"Data out of range\"\n-222,\"Data out of range\"\n-222,\"Data out of range\"\n-222,\"Data out of range\"\n-222,\"Data out of range\"\n-222,\"Data out of range\"\n-222,\"Data out of range\"\n-222,\"Data out of range\"\n-222,\"Data out of range\"\n-222,\"Data out of range\"\n-222,\"Data out of range\"\n-222,\"Data out of range\"\n-222,\"Data out of range\"\n-222,\"Data out of range\"\n-222,\"Data out of range\"\n-222,\"Data out of range\"\n-222,\"Data out of range\"\n-222,\"Data out of range\"\n-222,\"Data out of range\"\n-222,\"Data out of range\"\n-222,\"Data out of range\"\n-222,\"Data out of range\"\n-222,\"Data out of range\"\n-222,\"Data out of range\"\n-222,\"Data out of range\"\n-222,\"Data out of range\"\n-222,\"Data out of range\"\n-222,\"Data out of range\"\n-222,\"Data out of range\"\n-222,\"Data out of range\"\n-222,\"Data out of range\"\n-222,\"Data out of range\"\n-222,\"Data out of range\"\n-222,\"Data out of range\"\n-222,\"Data out of range\"\n-222,\"Data out of range\"\n-222,\"Data out of range\"\n-222,\"Data out of range\"\n-222,\"Data out of range\"\n-222,\"Data out of range\"\n-222,\"Data out of range\"\n-222,\"Data out of range\"\n-222,\"Data out of range\"\n-222,\"Data out of range\"\n-222,\"Data out of range\"\n-222,\"Data out of range\"\n-222,\"Data out of range\"\n-222,\"Data out of range\"\n-222,\"Data out of range\"\n-222,\"Data out of range\"\n-222,\"Data out of range\"\n-222,\"Data out of range\"\n-222,\"Data out of range\"\n-222,\"Data out of range\"\n-222,\"Data out of range\"\n-222,\"Data out of range\"\n-222,\"Data out of range\"\n-222,\"Data out of range\"\n-222,\"Data out of range\"\n-222,\"Data out of range\"\n-222,\"Data out of range\"\n-222,\"Data out of range\"\n-222,\"Data out of range\"\n-222,\"Data out of range\"\n-222,\"Data out of range\"\n-222,\"Data out of range\"\n-222,\"Data out of range\"\n-222,\"Data out of range\"\n-222,\"Data out of range\"\n-222,\"Data out of range\"\n-222,\"Data out of range\"\n-222,\"Data out of range\"\n-222,\"Data out of range\"\n-222,\"Data out of range\"\n-222,\"Data out of range\"\n-222,\"Data out of range\"\n-222,\"Data out of range\"\n-222,\"Data out of range\"\n-222,\"Data out of range\"\n-222,\"Data out of range\"\n-222,\"Data out of range\"\n-222,\"Data out of range\"\n-222,\"Data out of range\"\n-222,\"Data out of range\"\n-222,\"Data out of range\"\n-222,\"Data out of range\"\n-222,\"Data out of range\"\n-222,\"Data out of range\"\n-222,\"Data out of range\"\n-222,\"Data out of range\"\n-222,\"Data out of range\"\n-222,\"Data out of range\"\n-222,\"Data out of range\"\n-222,\"Data out of range\"\n-222,\"Data out of range\"\n-222,\"Data out of range\"\n-222,\"Data out of range\"\n-222,\"Data out of range\"\n-222,\"Data out of range\"\n-222,\"Data out of range\"\n"
  out "AUTO?":bool
  out "Zero Value":dbl format="%#.3p"
  out "Rng":string
  in  "Range":i16=1 min=1 max=6 step=1
  in  "Mono Port":refnum<visa-resource-name>="COM10"
  out "IDN String":string="Thorlabs,PM100USB,P2000362,1.3.0\n"
  out "Sensor SN":string="10061433"
  out "Sensor Name":string="S120C"
  out "Reply":string=" 0.000 nm  ok\r\n" caption="Mono Response"
  # "Range Settings"
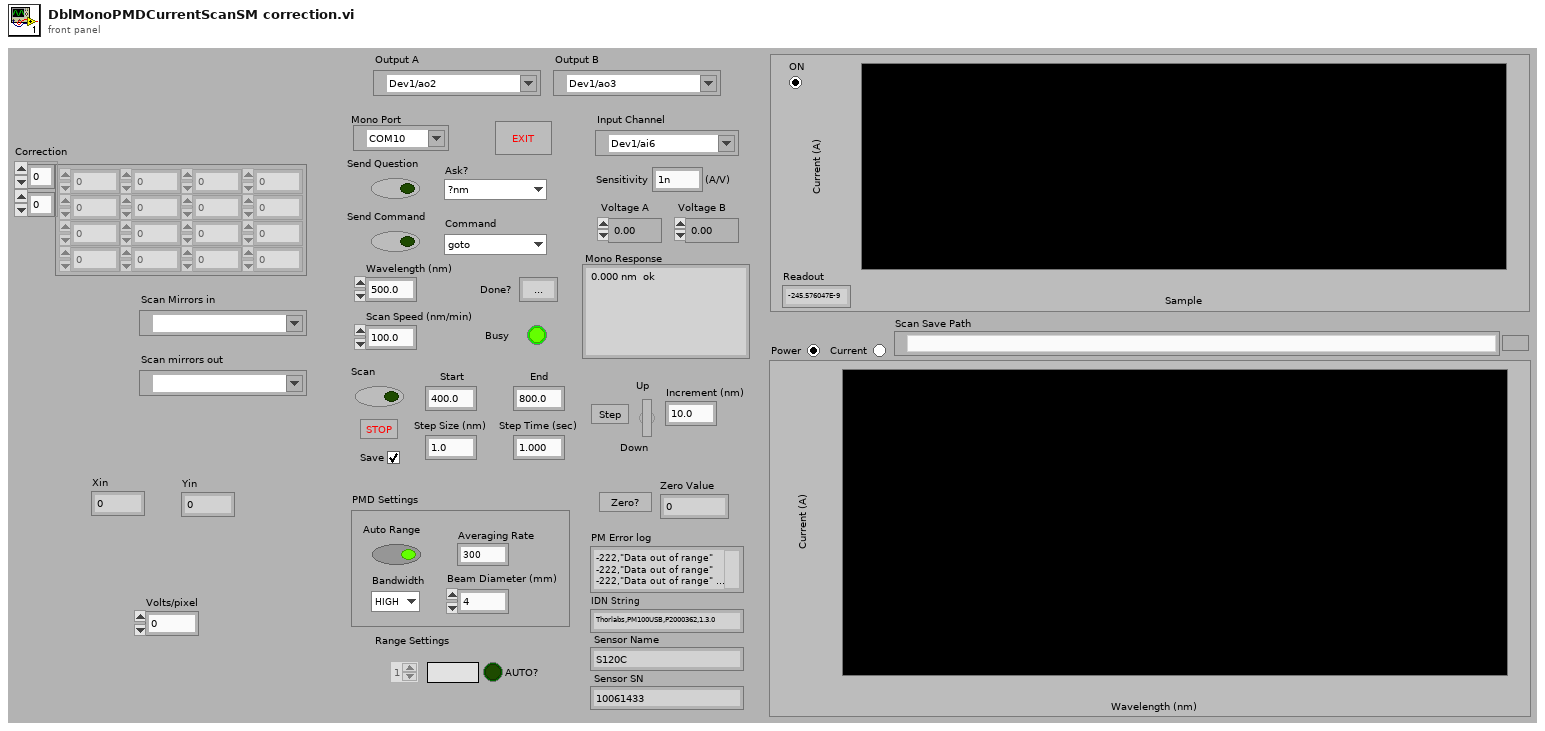
[diagram p1: front panel]
types:
  T1 = cluster{"Beam Diameter (mm)":dbl, "BWIn":u16, "Averaging Rate":i32, "Auto Range":bool}
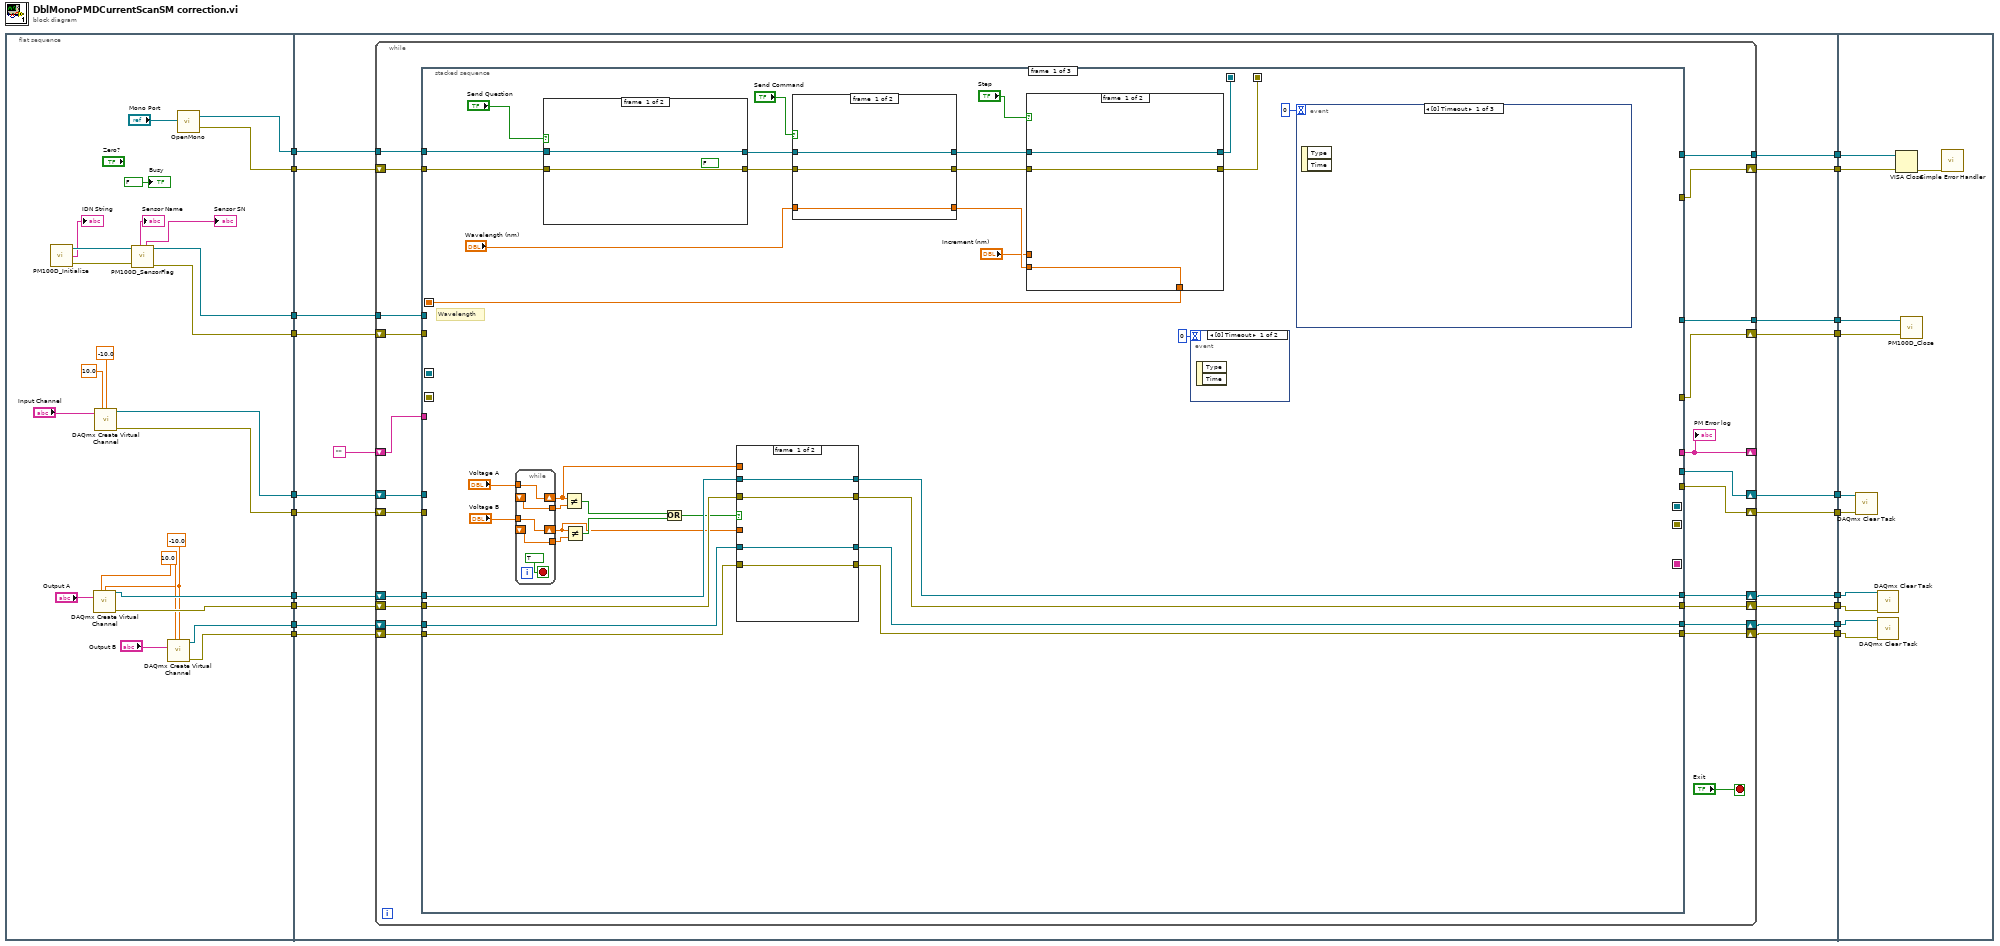
[diagram p0: block diagram]
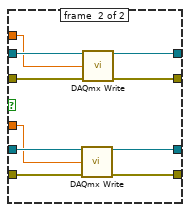
[diagram p2: hidden frame]
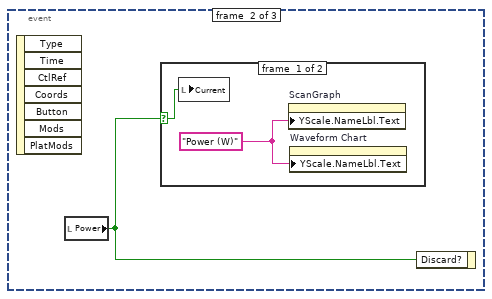
[diagram p3: hidden frame]
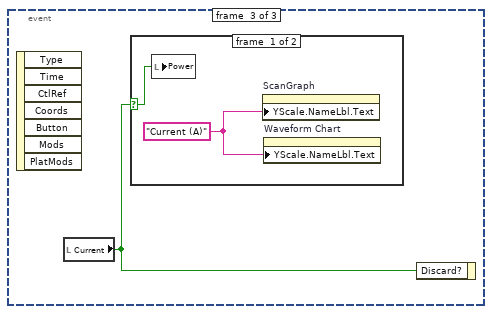
[diagram p5: hidden frame]
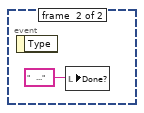
[diagram p7: hidden frame]
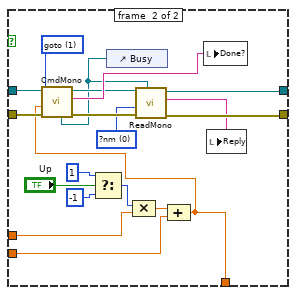
[diagram p8: hidden frame]
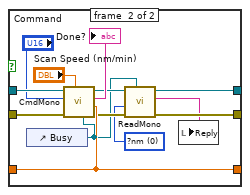
[diagram p9: hidden frame]
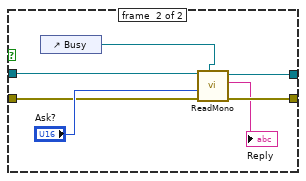
[diagram p10: hidden frame]
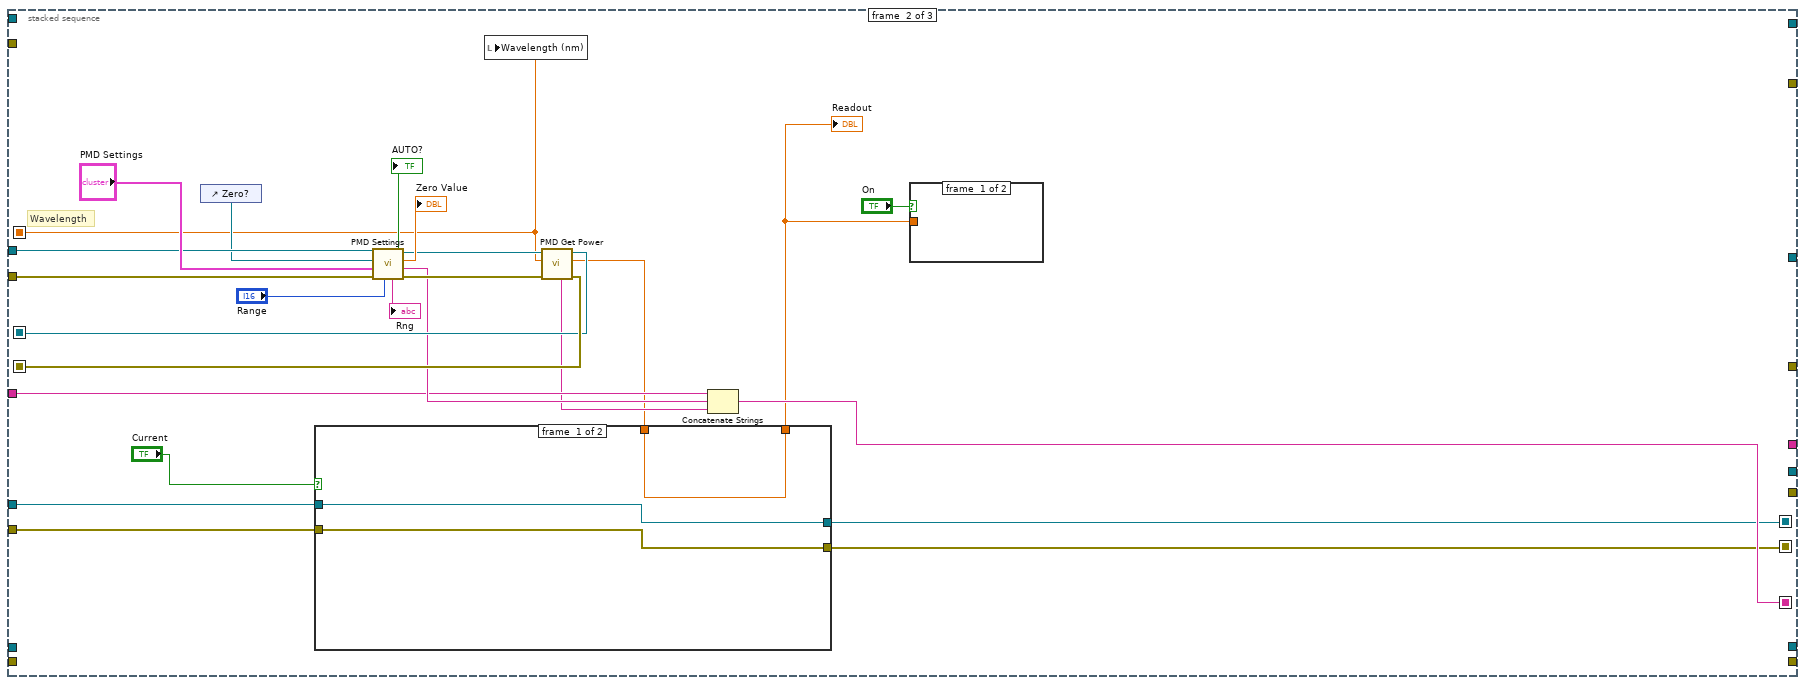
[diagram p11: hidden frame]
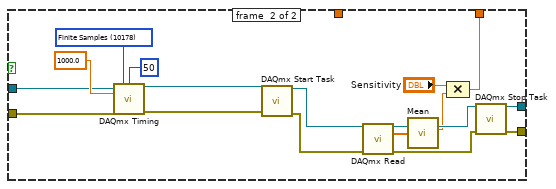
[diagram p12: hidden frame]
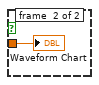
[diagram p13: hidden frame]
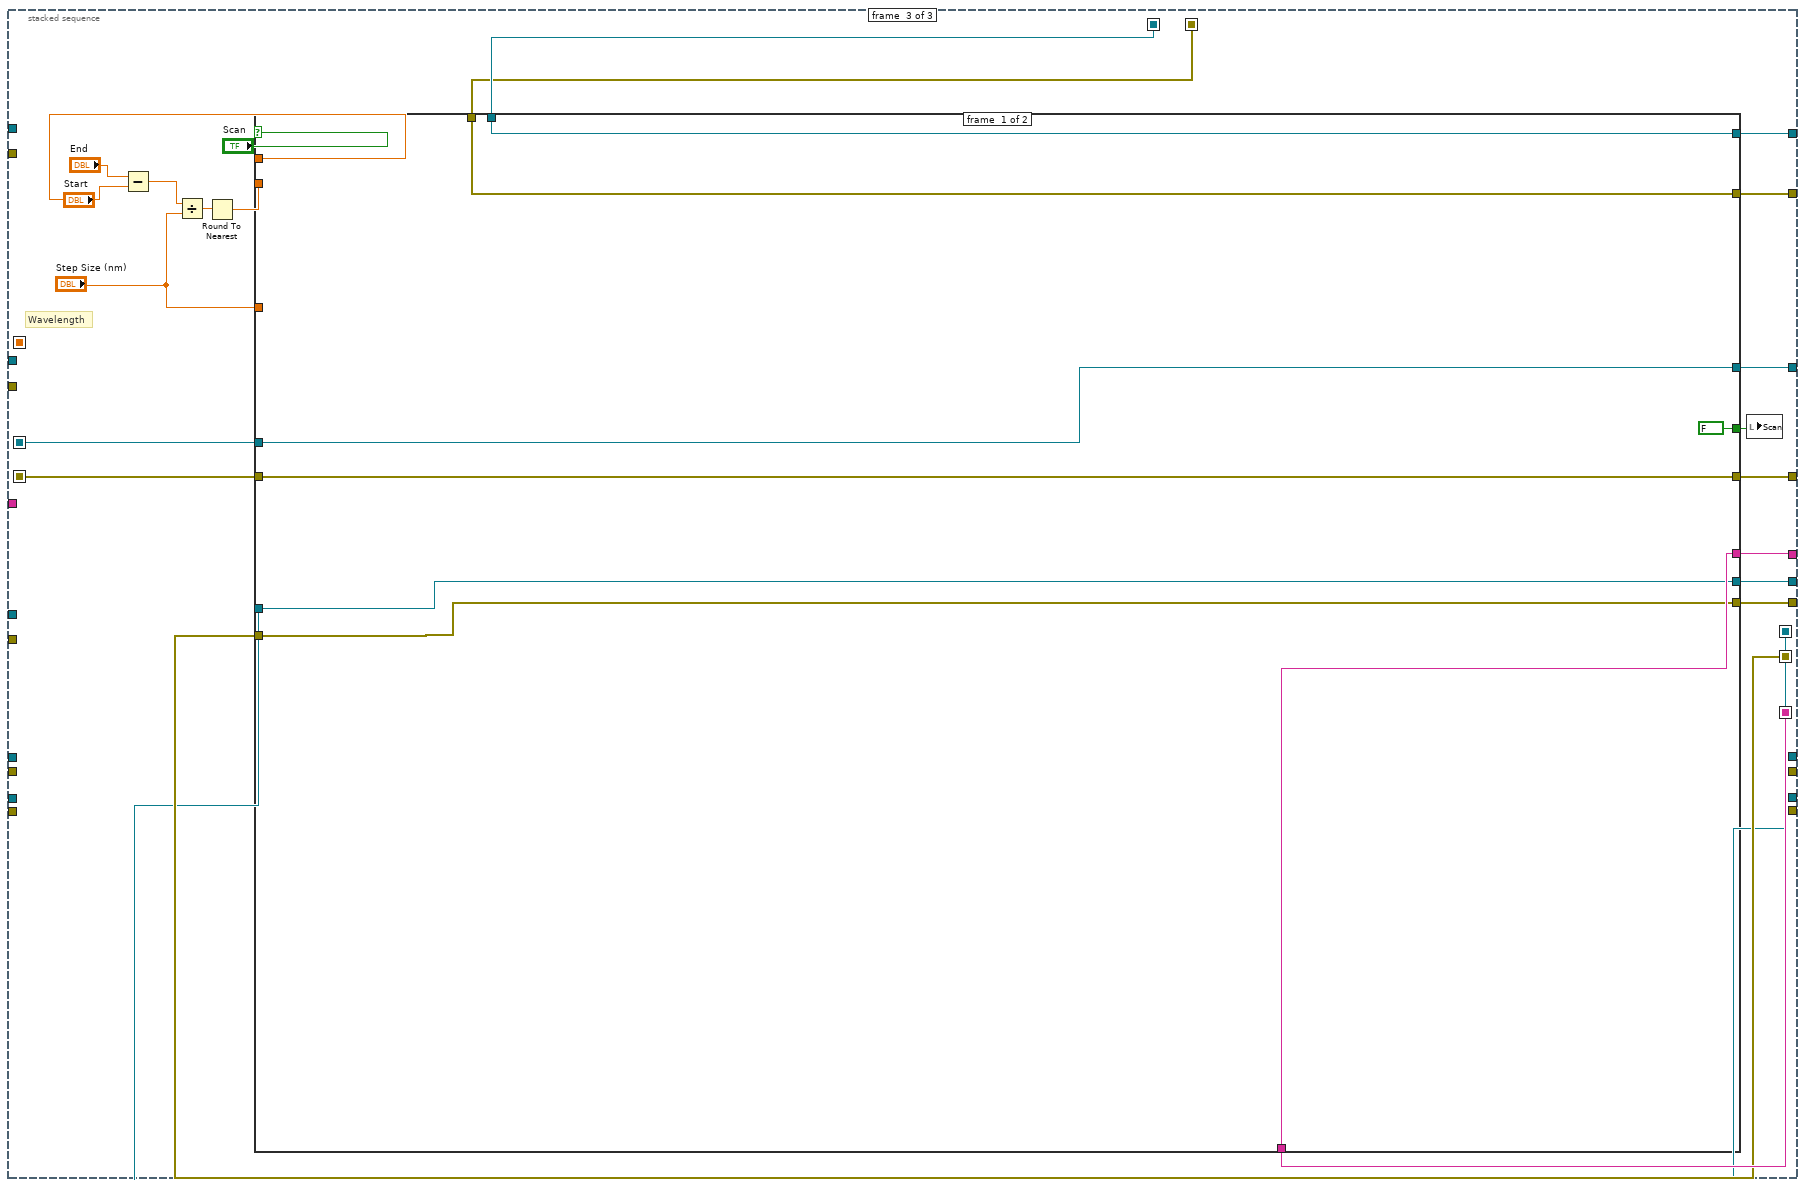
[diagram p14: hidden frame]
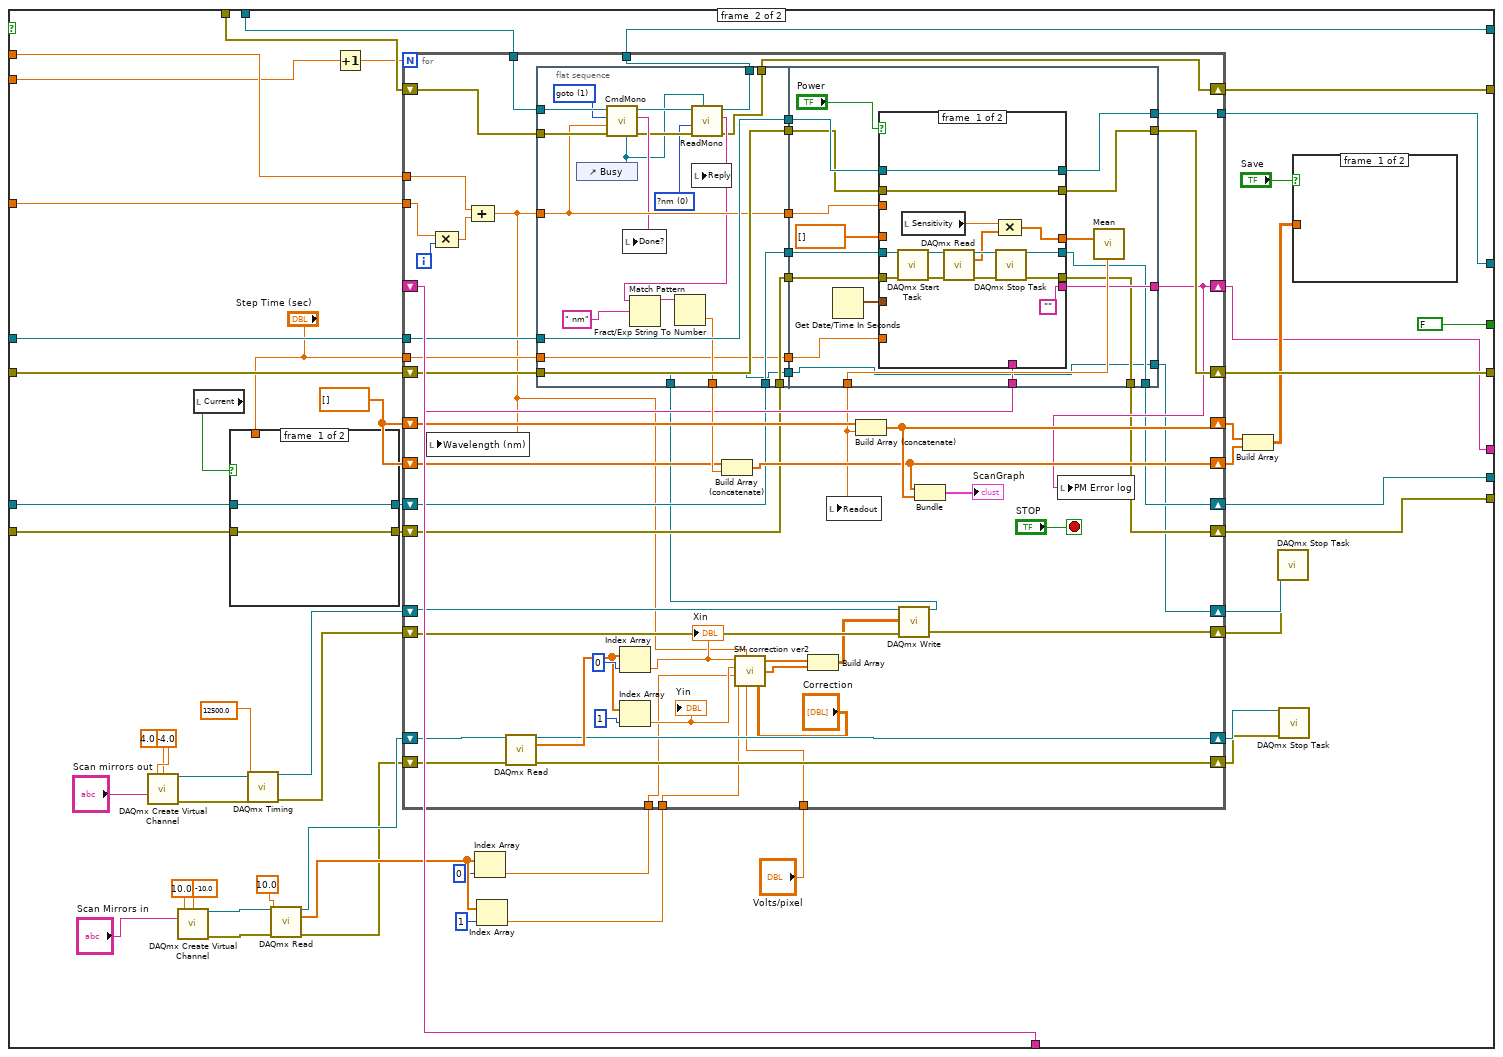
[diagram p15: hidden frame]
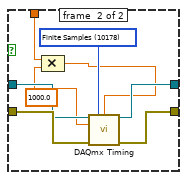
[diagram p16: hidden frame]
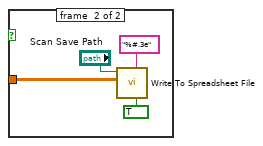
[diagram p17: hidden frame]
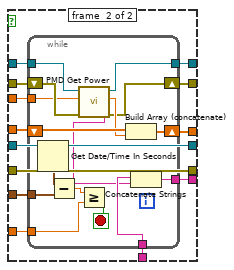
[diagram p18: hidden frame]
diagram:
  n1 = flat-sequence {
    tunnel: [w39] -> w20
    tunnel: [w38] -> w19
    tunnel: [w37] -> w18
    tunnel: [w36] -> w17
    tunnel: [w23] -> w12
    tunnel: [w24] -> w9
    tunnel: [w29] -> w8
    tunnel: [w30] -> w7
    tunnel: [w28] -> w6
    tunnel: [w27] -> w5
    tunnel: w20 -> [w64]
    tunnel: w19 -> [w65]
    tunnel: w18 -> [w63]
    tunnel: w17 -> [w62]
    tunnel: [w61] -> w16
    tunnel: [w60] -> w15
    tunnel: [w59] -> w14
    tunnel: [w58] -> w13
    tunnel: w12 -> [w55]
    tunnel: [w46] -> w11
    tunnel: [w45] -> w10
    tunnel: w9 -> [w56]
    tunnel: w8 -> [w54]
    tunnel: w7 -> [w53]
    tunnel: w6 -> [w52]
    tunnel: w5 -> [w51]
    tunnel: [w47] -> w4
    tunnel: [w48] -> w3
    tunnel: [w49] -> w2
    tunnel: [w50] -> w1
    tunnel: w16 -> [w487]
    tunnel: w15 -> [w486]
    tunnel: w14 -> [w485]
    tunnel: w13 -> [w484]
    tunnel: w11 -> [w482]
    tunnel: w10 -> [w483]
    tunnel: w4 -> [w481]
    tunnel: w3 -> [w480]
    tunnel: w2 -> [w479]
    tunnel: w1 -> [w478]
    frame #0 {
      w25 = -10.0 ("minimum value")
      w26 = 10.0 ("maximum value")
      n2 = call "PM100D_Initialize.vi"() -> ("error out"=w43:errorcluster, "Instrument"=→"IDN String":string, "VISA out"=w44:refnum<visa-resource-name>)  [unwired: 2 in, 1 out]
      n3 = call-poly <vilib>:"DAQmx Create Virtual Channel.vi"("maximum value"=w26, "minimum value"=w25, "physical channels"="Output A") -> ("task out"=w30:refnum<k21>, "error out"=w29:errorcluster)  [unwired: 11 in]
      n4 = call-poly <vilib>:"DAQmx Create Virtual Channel.vi"("maximum value"=10.0, "minimum value"=-10.0, "physical channels"="Input Channel") -> ("task out"=w24:refnum<k21>, "error out"=w23:errorcluster)  [unwired: 11 in]
      n5 = call "PM100D_SensorFlag.vi"("error in (no error)"=w43, "VISA in"=w44) -> ("error out"=w39:errorcluster, "VISA out"=w38:refnum<visa-resource-name>, "sn"=→"Sensor SN":string, "name"=→"Sensor Name":string)  [unwired: 2 in, 4 out]
      n6 = call-poly <vilib>:"DAQmx Create Virtual Channel.vi"("maximum value"=w26, "minimum value"=w25, "physical channels"="Output B") -> ("task out"=w27:refnum<k21>, "error out"=w28:errorcluster)  [unwired: 11 in]
      n7 = call "OpenMono.vi"("Mono Port"="Mono Port") -> ("VISA resource name out"=w37:refnum<visa-resource-name>, "error out"=w36:errorcluster)
      "Busy" <- FALSE ("Busy")
    }
    frame #1 {
      n8 = while {
        tunnel: w65 -> [w86]
        tunnel: w63 -> [w88]
        tunnel: [w83] -> w60
        tunnel: [w81] -> w58
        shift-right: [w80] -> w59
        shift-left: w64 -> [w85]
        shift-right: [w82] -> w61
        shift-left: w62 -> [w87]
        shift-right: [w78] -> _
        shift-left: "" -> [w79]
        shift-right: [w67] -> w45
        shift-left: w55 -> [w76]
        shift-right: [w66] -> w46
        shift-left: w56 -> [w77]
        shift-right: [w68] -> w50
        shift-left: w53 -> [w75]
        shift-right: [w69] -> w49
        shift-left: w54 -> [w74]
        shift-right: [w70] -> w48
        shift-left: w51 -> [w72]
        shift-right: [w71] -> w47
        shift-left: w52 -> [w73]
        stop <- "Exit" stop-if-true
        n9 = stacked-sequence {
          seq-local: [w107 _ _] -> [_ w203 _]
          seq-local: [w112 _ _] -> [_ _ w256]
          seq-local: [w111 _ _] -> [_ _ w255]
          seq-local: [_ w210 _] -> [_ _ w254]
          seq-local: [_ w211 _] -> [_ _ w253]
          seq-local: [_ w204 _] -> [_ _ w247]
          seq-local: [_ w198 _] -> [_ _ w243]
          seq-local: [_ w199 _] -> [_ _ w242]
          tunnel: w88 -> [w118 _ _]
          tunnel: w87 -> [w117 _ _]
          tunnel: w86 -> [_ w213 _]
          tunnel: w85 -> [_ w212 _]
          tunnel: [_ _ w252] -> w83
          tunnel: [_ _ w251] -> w82
          tunnel: [_ _ w250] -> w81
          tunnel: [_ _ w249] -> w80
          tunnel: w79 -> [_ w206 _]
          tunnel: [_ _ w246] -> w78
          tunnel: w77 -> [_ w197 _]
          tunnel: w76 -> [_ w196 _]
          tunnel: [_ _ w245] -> w66
          tunnel: [_ _ w244] -> w67
          tunnel: w75 -> [w102 _ _]
          tunnel: w74 -> [w103 _ _]
          tunnel: w73 -> [w105 _ _]
          tunnel: w72 -> [w104 _ _]
          tunnel: [w101 _ _] -> w71
          tunnel: [w100 _ _] -> w70
          tunnel: [w99 _ _] -> w69
          tunnel: [w98 _ _] -> w68
          frame #0 {
            # "Wavelength"
            n10 = while {
              shift-right: [w140] -> w89
              shift-left: _ -> [w139]
              tunnel: "Voltage B" -> [w140]
              tunnel: [w139] -> w94
              tunnel: "Voltage A" -> [w138]
              shift-right: [w138] -> w90
              shift-left: _ -> [w137]
              tunnel: [w137] -> w95
              stop <- TRUE stop-if-true
            }
            n11 = case shown="True" "Send Question" {
              tunnel: w118 -> [w188 w194]
              tunnel: w117 -> [w187 w193]
              tunnel: [w188 w192] -> w120
              tunnel: [w187 w191] -> w119
              frame #0 {
                (unwired) FALSE ("Read Error")
              }
              frame #1 {
                n12 = control-ref of="Busy"() -> (w189:refnum<vi>)
                n13 = call "ReadMono.vi"("Busy"=w189, "error in (no error)"=w193, "Cmd"="Ask?", "Mono Port"=w194) -> ("error out"=w191:errorcluster, "Response"=→"Reply":string, "Mono Port Out"=w192:refnum<visa-resource-name>)  [unwired: 2 in, 1 out]
              }
            }
            n14 = Not Equal?(x=w90, y=w95) -> (x != y?=w93:bool)
            n15 = Not Equal?(x=w89, y=w94) -> (x != y?=w92:bool)
            n16 = Or(x=w93, y=w92) -> (x .or. y?=w91:bool)
            n17 = case shown="True" w91 {
              tunnel: w105 -> [w123 w136]
              tunnel: w104 -> [w124 w135]
              tunnel: w103 -> [w125 w134]
              tunnel: w102 -> [w126 w133]
              tunnel: [w123 w132] -> w101
              tunnel: [w124 w131] -> w100
              tunnel: [w125 w130] -> w99
              tunnel: [w126 w129] -> w98
              tunnel: w90 -> [_ w127]
              tunnel: w89 -> [_ w128]
              frame #0 {
              }
              frame #1 {
                n18 = call-poly <vilib>:"DAQmx Write.vi"("task/channels in"=w135, "data"=w128, "error in"=w136) -> ("task out"=w131:refnum<k21>, "error out"=w132:errorcluster)  [unwired: 10 in, 1 out]
                n19 = call-poly <vilib>:"DAQmx Write.vi"("task/channels in"=w133, "data"=w127, "error in"=w134) -> ("task out"=w129:refnum<k21>, "error out"=w130:errorcluster)  [unwired: 10 in, 1 out]
              }
            }
            n20 = case shown="True" "Send Command" {
              tunnel: w120 -> [w173 w186]
              tunnel: w119 -> [w172 w185]
              tunnel: [w173 w178] -> w115
              tunnel: [w172 w177] -> w114
              tunnel: "Wavelength (nm)" -> [w171 w181]
              tunnel: [w171 w181] -> w113
              frame #0 {
              }
              frame #1 {
                w176 = u16 0 items=["?nm", "?nm/min", "?grating", "?turret", "?gratings"] ("Cmd")
                n21 = control-ref of="Busy"() -> (w174:refnum<vi>)
                n22 = call "CmdMono.vi"("Busy"=w174, "Scan Speed (nm/min)"="Scan Speed (nm/min)", "error in (no error)"=w185, "Wavelength (nm)"=w181, "Cmd"="Command", "Mono Port"=w186) -> ("error out"=w179:errorcluster, "Response"=→"Done?":string, "Mono Port Out"=w180:refnum<visa-resource-name>)  [unwired: 2 in, 1 out]
                n23 = call "ReadMono.vi"("Busy"=w174, "error in (no error)"=w179, "Cmd"=w176, "Mono Port"=w180) -> ("error out"=w177:errorcluster, "Response"=w175:string, "Mono Port Out"=w178:refnum<visa-resource-name>)  [unwired: 2 in, 1 out]
                n24 = local write "Reply"(w175) -> ()
              }
            }
            n25 = case shown="True" "Step" {
              tunnel: w115 -> [w151 w170]
              tunnel: w114 -> [w150 w169]
              tunnel: w113 -> [w149 w163]
              tunnel: [w151 w156] -> w112
              tunnel: [w150 w157] -> w111
              tunnel: "Increment (nm)" -> [_ w162]
              tunnel: [w149 w152] -> w107
              frame #0 {
              }
              frame #1 {
                w154 = u16 0 items=["?nm", "?nm/min", "?grating", "?turret", "?gratings"] ("Cmd")
                w161 = u16 1 items=["nm", "goto", "nm/min", "VIS grating", "IR grating"] ("Cmd")
                n26 = Select(t=1, s="Up", f=-1) -> (s? t:f=w168:i32)
                n27 = control-ref of="Busy"() -> (w153:refnum<vi>)
                n28 = Compound Arithmetic op=MULTIPLY(w168, w162) -> (w164:dbl)
                n29 = Compound Arithmetic op=ADD(w164, w163) -> (w152:dbl)
                n30 = call "CmdMono.vi"("Busy"=w153, "error in (no error)"=w169, "Wavelength (nm)"=w152, "Cmd"=w161, "Mono Port"=w170) -> ("error out"=w158:errorcluster, "Response"=w160:string, "Mono Port Out"=w159:refnum<visa-resource-name>)  [unwired: 3 in, 1 out]
                n31 = call "ReadMono.vi"("Busy"=w153, "error in (no error)"=w158, "Cmd"=w154, "Mono Port"=w159) -> ("error out"=w157:errorcluster, "Response"=w155:string, "Mono Port Out"=w156:refnum<visa-resource-name>)  [unwired: 2 in, 1 out]
                n32 = local write "Done?"(w160) -> ()
                n33 = local write "Reply"(w155) -> ()
              }
            }
            n34 = event shown="[0] Timeout" {
              selector: _ -> [_ _]
              dyn-events: _ -> [_ _]
              timeout: 0 -> [_ _]
              event #0 {
                n35 = event-data() -> ()  [unwired: 1 in, 2 out]
              }
              event #1 {
                n36 = event-data() -> ()  [unwired: 1 in, 1 out]
                n37 = local write "Done?"("   ..." ("Done?")) -> ()
              }
            }
            n38 = event shown="[0] Timeout" {
              selector: _ -> [_ _ _]
              dyn-events: _ -> [_ _ _]
              timeout: 0 -> [_ _ _]
              event #0 {
                n39 = event-data() -> ()  [unwired: 1 in, 2 out]
              }
              event #1 {
                n40 = event-data() -> ()  [unwired: 1 in, 7 out]
                n41 = local read "Power"() -> (w142:bool)
                n42 = case shown="False" w142 {
                  selector: w142 -> [w144 _]
                  frame #0 {
                    w143 = "Power (W)" ("Y Scale.Name Label.Text")
                    n43 = local write "Current"(w144) -> ()
                    n44 = property on="ScanGraph" class="XYGraph (strict)"("YScale.NameLbl.Text"=w143) -> ()  [unwired: 2 in, 2 out]
                    n45 = property on="Waveform Chart" class="WFChart (strict)"("YScale.NameLbl.Text"=w143) -> ()  [unwired: 2 in, 2 out]
                  }
                  frame #1 {
                  }
                }
                n46 = event-data("Discard?"=w142) -> ()  [unwired: 1 in, 1 out]
              }
              event #2 {
                n47 = event-data() -> ()  [unwired: 1 in, 7 out]
                n48 = local read "Current"() -> (w145:bool)
                n49 = case shown="False" w145 {
                  selector: w145 -> [w146 _]
                  frame #0 {
                    w147 = "Current (A)" ("Y Scale.Name Label.Text")
                    n50 = local write "Power"(w146) -> ()
                    n51 = property on="ScanGraph" class="XYGraph (strict)"("YScale.NameLbl.Text"=w147) -> ()  [unwired: 2 in, 2 out]
                    n52 = property on="Waveform Chart" class="WFChart (strict)"("YScale.NameLbl.Text"=w147) -> ()  [unwired: 2 in, 2 out]
                  }
                  frame #1 {
                  }
                }
                n53 = event-data("Discard?"=w145) -> ()  [unwired: 1 in, 1 out]
              }
            }
          }
          frame #1 {
            # "Wavelength"
            n54 = control-ref of="Zero?"() -> (w208:refnum<vi>)
            n55 = call "PMD Settings.vi"("Visa In"=w213, "Zero?"=w208, "PMD Settings In"="PMD Settings", "Error In"=w212, "Range"="Range") -> ("AUTO?"=→"AUTO?":bool, "Rng"=→"Rng":string, "Visa Out"=w216:refnum<visa-resource-name>, "ZeroValue"=→"Zero Value":dbl, "PM Error log"=w207:string, "error out"=w215:errorcluster)
            n56 = local write "Wavelength (nm)"(w203) -> ()
            n57 = call "PMD Get Power.vi"("VISA In"=w216, "Wavelength (nm)"=w203, "error in"=w215) -> ("PMD Error"=w205:string, "VISA out"=w210:refnum<visa-resource-name>, "Readout value"=w202:dbl, "error out"=w211:errorcluster)  [unwired: 1 in, 2 out]
            n58 = case shown="False" "Current" {
              tunnel: w202 -> [w223 _]
              tunnel: w197 -> [w222 w226]
              tunnel: w196 -> [w221 w227]
              tunnel: [w223 w239] -> w200
              tunnel: [w221 w235] -> w198
              tunnel: [w222 w236] -> w199
              frame #0 {
              }
              frame #1 {
                w229 = 10178 items=["Finite Samples"=10178, "Continuous Samples"=10123, "Hardware Timed Single Point"=12522] ("sample mode")
                n59 = call-poly <vilib>:"DAQmx Timing.vi"("task/channels in"=w226, "sample mode"=w229, "samples per channel"=50, "rate"=1000.0, "error in"=w227) -> ("task out"=w225:refnum<k21>, "error out"=w224:errorcluster)  [unwired: 9 in]
                n60 = call <vilib>:"DAQmx Start Task.vi"("task/channels in"=w225, "error in"=w224) -> ("task out"=w237:refnum<k21>, "error out"=w238:errorcluster)  [unwired: 12 in]
                n61 = call-poly <vilib>:"DAQmx Read.vi"("task/channels in"=w237, "error in"=w238) -> ("task out"=w233:refnum<k21>, "data"=w232:dbl[], "error out"=w234:errorcluster)  [unwired: 11 in]
                n62 = call <vilib>:"Mean.vi"("X"=w232) -> ("mean"=w231:dbl)  [unwired: 1 out]
                n63 = Compound Arithmetic op=MULTIPLY("Sensitivity", w231) -> (w239:dbl)
                n64 = call <vilib>:"DAQmx Stop Task.vi"("task/channels in"=w233, "error in"=w234) -> ("task out"=w236:refnum<k21>, "error out"=w235:errorcluster)  [unwired: 12 in]
              }
            }
            "Readout" <- w200
            n65 = Concatenate Strings(w206, w207, w205) -> (w204:string)
            n66 = case shown="True" "On" {
              tunnel: w200 -> [_ w241]
              frame #0 {
              }
              frame #1 {
                "Waveform Chart" <- w241
              }
            }
          }
          frame #2 {
            # "Wavelength"
            n67 = Subtract(x="End", y="Start") -> (x-y=w261:dbl)
            n68 = Divide(x=w261, y="Step Size (nm)") -> (x/y=w260:dbl)
            n69 = Round To Nearest(number=w260) -> (nearest integer value=w259:dbl)
            n70 = case shown="True" "Scan" {
              tunnel: w259 -> [_ w320]
              tunnel: w255 -> [w269 w322]
              tunnel: w256 -> [w268 w323]
              tunnel: "Start" -> [_ w325]
              tunnel: "Step Size (nm)" -> [_ w324]
              tunnel: w254 -> [w271 w318]
              tunnel: w253 -> [w270 w317]
              tunnel: [w271 w306] -> w250
              tunnel: [w270 w316] -> w249
              tunnel: [w269 w315] -> w251
              tunnel: [w268 w314] -> w252
              tunnel: [FALSE ("Scan") FALSE ("Scan")] -> w248
              tunnel: w247 -> [w266 w308]
              tunnel: [w266 w307] -> w246
              tunnel: [w265 w305] -> w245
              tunnel: [w264 w304] -> w244
              tunnel: w243 -> [w264 w302]
              tunnel: w242 -> [w265 w301]
              frame #0 {
              }
              frame #1 {
                w321 = dbl[] []
                n71 = call-poly <vilib>:"DAQmx Create Virtual Channel.vi"("maximum value"=-4.0, "minimum value"=4.0, "physical channels"="Scan mirrors out") -> ("task out"=w281:refnum<k21>, "error out"=w279:errorcluster)  [unwired: 11 in]
                n72 = call-poly <vilib>:"DAQmx Create Virtual Channel.vi"("maximum value"=10.0, "minimum value"=-10.0, "physical channels"="Scan Mirrors in") -> ("task out"=w292:refnum<k21>, "error out"=w296:errorcluster)  [unwired: 11 in]
                n73 = local read "Current"() -> (w303:bool)
                n74 = case shown="True" w303 {
                  tunnel: w302 -> [w326 w334]
                  tunnel: w301 -> [w327 w333]
                  tunnel: [w327 w332] -> w300
                  tunnel: [w326 w331] -> w299
                  tunnel: "Step Time (sec)" -> [_ w330]
                  frame #0 {
                  }
                  frame #1 {
                    w335 = 10178 items=["Finite Samples"=10178, "Continuous Samples"=10123, "Hardware Timed Single Point"=12522] ("sample mode")
                    w329 = 1000.0 ("rate")
                    n75 = Compound Arithmetic op=MULTIPLY(w330, w329) -> (w328:dbl)
                    n76 = call-poly <vilib>:"DAQmx Timing.vi"("task/channels in"=w333, "sample mode"=w335, "samples per channel"=w328, "rate"=w329, "error in"=w334) -> ("task out"=w332:refnum<k21>, "error out"=w331:errorcluster)  [unwired: 9 in]
                  }
                }
                n77 = call-poly <vilib>:"DAQmx Timing.vi"("task/channels in"=w281, "rate"=12500.0, "error in"=w279) -> ("task out"=w280:refnum<k21>, "error out"=w278:errorcluster)  [unwired: 11 in]
                n78 = call-poly <vilib>:"DAQmx Read.vi"("task/channels in"=w292, "timeout"=10.0, "error in"=w296) -> ("task out"=w277:refnum<k21>, "data"=w291:dbl[], "error out"=w276:errorcluster)  [unwired: 10 in]
                n79 = Increment(x=w320) -> (x+1=w319:dbl)
                n80 = Index Array(array=w291, index=0) -> (element=w288:dbl)
                n81 = Index Array(array=w291, index=1) -> (element=w287:dbl)
                n82 = for {
                  N: w319 -> [_]
                  tunnel: w323 -> [w393]
                  tunnel: w325 -> [w389]
                  tunnel: w324 -> [w391]
                  shift-right: [w377] -> w313
                  shift-left: w321 -> [w395]
                  shift-right: [w388] -> w315
                  shift-left: w322 -> [w394]
                  shift-right: [w374] -> w312
                  shift-left: w321 -> [w375]
                  tunnel: w318 -> [w386]
                  shift-right: [w381] -> w316
                  shift-left: w317 -> [w385]
                  tunnel: [w380] -> w306
                  tunnel: [w379] -> w314
                  shift-right: [w372] -> w307
                  shift-left: w308 -> [w373]
                  shift-right: [w369] -> w304
                  shift-left: w299 -> [w364]
                  shift-right: [w368] -> w305
                  shift-left: w300 -> [w365]
                  tunnel: "Step Time (sec)" -> [w366]
                  tunnel: w288 -> [w349]
                  tunnel: w287 -> [w348]
                  shift-right: [w343] -> w283
                  shift-left: w280 -> [w362]
                  shift-right: [w356] -> w282
                  shift-left: w278 -> [w361]
                  shift-right: [w355] -> w275
                  shift-left: w277 -> [w354]
                  shift-right: [w352] -> w274
                  shift-left: w276 -> [w353]
                  tunnel: "Volts/pixel" -> [w340]
                  i -> [w392]
                  stop <- "STOP" stop-if-true
                  n83 = Compound Arithmetic op=MULTIPLY(w391, w392) -> (w390:dbl)
                  n84 = Compound Arithmetic op=ADD(w389, w390) -> (w347:dbl)
                  n85 = local write "Wavelength (nm)"(w347) -> ()
                  n86 = call-poly <vilib>:"DAQmx Read.vi"("task/channels in"=w354, "error in"=w353) -> ("task out"=w355:refnum<k21>, "data"=w358:dbl[], "error out"=w352:errorcluster)  [unwired: 11 in]
                  n87 = flat-sequence {
                    tunnel: w394 -> [w416]
                    tunnel: w393 -> [w415]
                    tunnel: w347 -> [w411]
                    tunnel: [w400] -> w388
                    tunnel: w386 -> [w413]
                    tunnel: w385 -> [w412]
                    tunnel: [w413] -> w384
                    tunnel: [w412] -> w383
                    tunnel: [w411] -> w382
                    tunnel: [w405] -> w379
                    tunnel: [w401] -> w376
                    tunnel: w364 -> [w398]
                    tunnel: [w399] -> w371
                    tunnel: w365 -> [w399]
                    tunnel: [w398] -> w370
                    tunnel: [w397] -> w367
                    tunnel: w366 -> [w397]
                    tunnel: w342 -> [w396]
                    tunnel: [w396] -> w341
                    tunnel: [w431] -> w363
                    tunnel: w384 -> [w430]
                    tunnel: w383 -> [w429]
                    tunnel: w382 -> [w428]
                    tunnel: [w424] -> w381
                    tunnel: [w427] -> w380
                    tunnel: w373 -> [w426]
                    tunnel: [w425] -> w372
                    tunnel: w371 -> [w422]
                    tunnel: w370 -> [w421]
                    tunnel: [w419] -> w368
                    tunnel: [w420] -> w369
                    tunnel: w367 -> [w423]
                    tunnel: [w417] -> w343
                    tunnel: w341 -> [w417]
                    frame #0 {
                      w407 = u16 0 items=["?nm", "?nm/min", "?grating", "?turret", "?gratings"] ("Cmd")
                      w414 = u16 1 items=["nm", "goto", "nm/min", "VIS grating", "IR grating"] ("Cmd")
                      n88 = control-ref of="Busy"() -> (w406:refnum<vi>)
                      n89 = call "CmdMono.vi"("Busy"=w406, "error in (no error)"=w416, "Wavelength (nm)"=w411, "Cmd"=w414, "Mono Port"=w415) -> ("error out"=w408:errorcluster, "Response"=w410:string, "Mono Port Out"=w409:refnum<visa-resource-name>)  [unwired: 3 in, 1 out]
                      n90 = local write "Done?"(w410) -> ()
                      n91 = call "ReadMono.vi"("Busy"=w406, "error in (no error)"=w408, "Cmd"=w407, "Mono Port"=w409) -> ("error out"=w400:errorcluster, "Response"=w403:string, "Mono Port Out"=w405:refnum<visa-resource-name>)  [unwired: 2 in, 1 out]
                      n92 = Match Pattern(string=w403, regular expression=" nm") -> (before substring=w402:string)  [unwired: 1 in, 3 out]
                      n93 = Fract/Exp String To Number(string=w402) -> (number=w401:dbl)  [unwired: 3 in, 1 out]
                      n94 = local write "Reply"(w403) -> ()
                    }
                    frame #1 {
                      n95 = Get Date/Time In Seconds() -> (seconds since 1Jan1904=w433:timestamp)
                      n96 = case shown="False" "Power" {
                        tunnel: dbl[] [] -> [_ w461]
                        tunnel: w433 -> [_ w460]
                        tunnel: [w435 w459] -> w432
                        tunnel: w430 -> [w447 w458]
                        tunnel: w429 -> [w446 w457]
                        tunnel: w428 -> [_ w456]
                        tunnel: [w447 w455] -> w427
                        tunnel: w426 -> [_ w454]
                        tunnel: ["" w453] -> w425
                        tunnel: [w446 w452] -> w424
                        tunnel: w423 -> [_ w451]
                        tunnel: w422 -> [w445 w449]
                        tunnel: w421 -> [w444 w450]
                        tunnel: [w439 w450] -> w420
                        tunnel: [w438 w449] -> w419
                        frame #0 {
                          n97 = call <vilib>:"DAQmx Start Task.vi"("task/channels in"=w445, "error in"=w444) -> ("task out"=w443:refnum<k21>, "error out"=w442:errorcluster)  [unwired: 12 in]
                          n98 = local read "Sensitivity"() -> (w436:dbl)
                          n99 = call-poly <vilib>:"DAQmx Read.vi"("task/channels in"=w443, "error in"=w442) -> ("task out"=w441:refnum<k21>, "data"=w437:dbl[], "error out"=w440:errorcluster)  [unwired: 11 in]
                          n100 = call <vilib>:"DAQmx Stop Task.vi"("task/channels in"=w441, "error in"=w440) -> ("task out"=w438:refnum<k21>, "error out"=w439:errorcluster)  [unwired: 12 in]
                          n101 = Compound Arithmetic op=MULTIPLY(w436, w437) -> (w435:dbl[])
                        }
                        frame #1 {
                          n102 = while {
                            shift-right: [w476] -> w459
                            shift-left: w461 -> [w477]
                            tunnel: w460 -> [w474]
                            tunnel: w458 -> [w469]
                            tunnel: w456 -> [w465]
                            tunnel: [w467] -> w455
                            tunnel: w454 -> [w471]
                            tunnel: [w470] -> w453
                            shift-right: [w463] -> w452
                            shift-left: w457 -> [w468]
                            tunnel: w451 -> [w462]
                            stop <- w472 stop-if-true
                            n103 = Get Date/Time In Seconds() -> (seconds since 1Jan1904=w475:timestamp)
                            n104 = Subtract(x=w475, y=w474) -> (x-y=w473:dbl)
                            n105 = call "PMD Get Power.vi"("VISA In"=w469, "Wavelength (nm)"=w465, "error in"=w468) -> ("PMD Error"=w464:string, "VISA out"=w467:refnum<visa-resource-name>, "Readout value"=w466:dbl, "error out"=w463:errorcluster)  [unwired: 1 in, 2 out]
                            n106 = Greater Or Equal?(x=w473, y=w462) -> (x >= y?=w472:bool)
                            n107 = Build Array (concatenate)(w477, w466) -> (w476:dbl[])
                            n108 = Concatenate Strings(w471, w464) -> (w470:string)
                          }
                        }
                      }
                      n109 = call <vilib>:"Mean.vi"("X"=w432) -> ("mean"=w431:dbl)  [unwired: 1 out]
                    }
                  }
                  n110 = Index Array(array=w358, index=0) -> (element=w351:dbl)
                  "Xin" <- w351
                  n111 = Index Array(array=w358, index=1) -> (element=w350:dbl)
                  "Yin" <- w350
                  n112 = Build Array (concatenate)(w375, w376) -> (w374:dbl[])
                  n113 = call "SM correction ver2.vi"("V in x"=w351, "nm in"=w347, "V in y"=w350, "V x initial"=w349, "Volts/pixel"=w340, "V y initial"=w348, "Array"="Correction") -> ("V out x"=w346:dbl[], "V out y"=w345:dbl[])
                  n114 = Build Array(w346, w345) -> (w357:dbl[][])
                  n115 = local write "Readout"(w363) -> ()
                  n116 = Build Array (concatenate)(w395, w363) -> (w377:dbl[])
                  n117 = call-poly <vilib>:"DAQmx Write.vi"("task/channels in"=w362, "data"=w357, "error in"=w361) -> ("task out"=w342:refnum<k21>, "error out"=w356:errorcluster)  [unwired: 10 in, 1 out]
                  n118 = Bundle(w374, w377) -> (→"ScanGraph":cluster{dbl[], dbl[]})  [unwired: 1 in]
                  n119 = local write "PM Error log"(w372) -> ()
                }
                n120 = Build Array(w313, w312) -> (w311:dbl[][])
                n121 = call <vilib>:"DAQmx Stop Task.vi"("task/channels in"=w283, "error in"=w282) -> ()  [unwired: 12 in, 2 out]
                n122 = call <vilib>:"DAQmx Stop Task.vi"("task/channels in"=w275, "error in"=w274) -> ()  [unwired: 12 in, 2 out]
                n123 = case shown="True" "Save" {
                  tunnel: w311 -> [_ w336]
                  frame #0 {
                  }
                  frame #1 {
                    n124 = call-poly <vilib>:"Write To Spreadsheet File.vi"("transpose? (no:F)"=TRUE, "format (%.3f)"="%#.3e", "2D data"=w336, "file path (dialog if empty)"="Scan Save Path") -> ()  [unwired: 4 in, 1 out]
                  }
                }
              }
            }
            n125 = local write "Scan"(w248) -> ()
          }
        }
        "PM Error log" <- w78
      }
    }
    frame #2 {
      n126 = call <vilib>:"DAQmx Clear Task.vi"("task in"=w482, "error in"=w483) -> ()  [unwired: 13 in, 1 out]
      n127 = call <vilib>:"DAQmx Clear Task.vi"("task in"=w478, "error in"=w479) -> ()  [unwired: 13 in, 1 out]
      n128 = call <vilib>:"DAQmx Clear Task.vi"("task in"=w480, "error in"=w481) -> ()  [unwired: 13 in, 1 out]
      n129 = VISA Close(VISA resource name=w486, error in (no error)=w487) -> (error out=w488:errorcluster)
      n130 = call "PM100D_Close.vi"("error in (no error)"=w485, "VISA resource name"=w484) -> ()  [unwired: 2 in]
      n131 = call <vilib>:"Simple Error Handler.vi"("error in (no error)"=w488) -> ()  [unwired: 1 in, 8 out]
    }
  }
